vi "Measurement.vi"(0 "Position":T3(array[cluster]) {"Z" format="%.1f"; "Y" format="%.1f"; "X" format="%.1f"}, 1 "setup":T4=enum."Show Setup", 2 "Post Process":T2, 4 "File":T5, 5 "Results file":path, 7 "Raw data file":path, 11 "Setup filename":string) -> (14 "2nd plot":cluster{"X array":dbl[], "Y array":dbl[]}[](graph), 19 "Status Out":T1)   [LabVIEW 2013]
uses:
  Anemometry Sub Vis/Controls/Save_Data.ctl
  Anemometry Sub Vis/Controls/Setup.ctl
  Anemometry Sub Vis/Controls/Graph_Type.ctl
  Anemometry Sub Vis/Controls/Post_Process.ctl
  Anemometry Sub Vis/Gen Trav/Multi_Run_Status.ctl
  Anemometry Sub Vis/Controls/Inst_type.ctl
  ADAM Client/Sub VIs/ADAM Controls/Traverse_Level_State.ctl
  Anemometry Sub Vis/File/Setup_Filetype.ctl
  Anemometry Sub Vis/Globals/Trav_pos_global.vi
  Anemometry Sub Vis/Globals/Meas_global.vi
  Anemometry Sub Vis/Acquisition/PWA/PWAtasksGLOBAL.vi
  Anemometry Sub Vis/Acquisition/Data_Translation/DataTranslation_global.vi
  Anemometry Sub Vis/Globals/Preference_global.vi
  Anemometry Sub Vis/Globals/LDA_meas_global_1.vi
  Anemometry Sub Vis/Globals/LDA_meas_global_2.vi
  Anemometry Sub Vis/Globals/Dynamic_call_global.ph.vi
  Anemometry Sub Vis/Globals/Plug_in_data_global.vi
  Anemometry Sub Vis/Globals/Constants_global.vi
panel:
  out "Pause message":string
  out "Statistics":string[][](table)
  out "Actual Sampling freq":dbl=100.0 format="%.1f"
  in  "Desired Sampling freq (Hz)":dbl=100.0 format="%.1f"
  out "Current Block No":i32=5 caption="Current Block"
  in  "Pause":bool
  in  "No of Blocks":i32=5
  in  "stop":bool
  in  "No of samples":i32=1000 min=0 step=1
  in  "PP next block":bool
  in  "Tab Control":T6(tab)
  in  "Second Graph":T8={"Plot 1"=2, "Plot 2"=1, "Save graph"=0, "Plot Type"=enum."Vel histogram"} {"Save graph" items=["Do not save plot", "Save plot"]; "Plot 2" items=["Nothing", "U1", "U2", "Sync", "T", "WT1", "I1"]; "Plot 1" items=["Nothing", "U1", "U2", "Sync", "T", "WT1", "I1"]}
  in  "First Graph":T8={"Plot 1"=1, "Plot 2"=2, "Save graph"=0, "Plot Type"=enum."Velocity trace"} {"Save graph" items=["Do not save plot", "Save plot"]; "Plot 2" items=["Nothing", "U1", "U2", "Sync", "T", "WT1", "I1"]; "Plot 1" items=["Nothing", "U1", "U2", "Sync", "T", "WT1", "I1"]}
  out "First plot":cluster{"X array":dbl[], "Y array":dbl[]}[](graph)
  in  "Comments":string
  out "uv":dbl[][](graph)=[[-0.041806189081711534, -0.046435429052714985, -0.04035660097427599, -0.042187605126076694, -0.042052555599004206]]
  out "u^4":dbl[][](graph)
  out "u^3":dbl[][](graph)
  out "u^2":dbl[][](graph)=[[0.09743628875280319, 0.10575821456272283, 0.10126262927293661, 0.09890442087602569, 0.1022948212436432]]
  out "U":dbl[][](graph)=[[0.8295029456391334, 0.8915896983798417, 0.8415763502225625, 0.8394746126219594, 0.8466062785395404]]
  in  "Block average display control":cluster{"Name":string, "Include":bool}[](array[cluster])=[{"Name"="FF (C)", "Include"=FALSE}]
  in  "No of bins in histogram":i32=100
  out "Measurement time (min)":dbl=6.0 format="%.2f"
  in  "Correlate?":T9(ring)
  out "Diagnostic info":string[][](table)
  out "Array U":dbl[][](array[numeric]) format="%.2e"
  out "Array u^2":dbl[][](array[numeric]) format="%.2e"
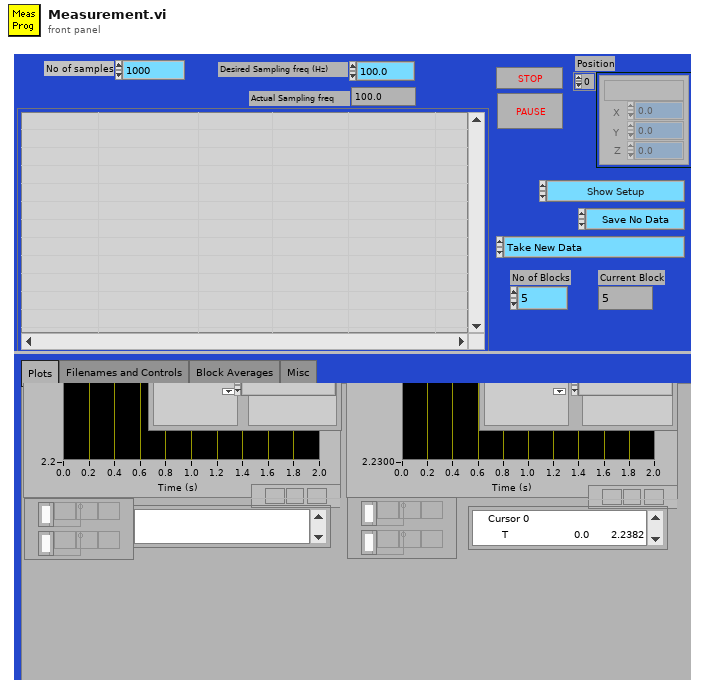
[diagram p1: front panel]
types:
  T1 = typedef "Multi_Run_Status.ctl" = enum16{"Continue", "Jump to Next Point", "Jump to Next Row", "Jump To Fall Back", "Terminate Run"}
  T2 = typedef "Post_Process.ctl" = enum16{"Take New Data", "Post Process Raw Data File"}
  T3 = cluster{"Name":string, "X":dbl, "Y":dbl, "Z":dbl}[]
  T4 = typedef "Setup.ctl" = enum16{"Run Program", "Show Setup", "Save Current Setup", "Setup Front Panel"}
  T5 = typedef "Save_Data.ctl" = enum16{"Save No Data", "Save Data"}
  T6 = enum32{"Plots", "Filenames and Controls", "Block Averages", "Misc"}
  T7 = typedef "Graph_Type.ctl" = enum16{"Show no graph", "Voltage trace", "Velocity trace", "Vel histogram", "Spectrum", "f.E(f) v Log f", "Auto-Corr"}
  T8 = cluster{"Plot 1":u16, "Plot 2":u16, "Save graph":u16, "Plot Type":T7}
  T9 = enum16{"Cross correlation off", "Show correlation panel", "Correlate without activating panel"}
  T10 = enum32{"Bad", "Idle", "Run top level", "Running"}
  T11 = cluster{"Name":string, "X":dbl, "Y":dbl, "Z":dbl}
  T12 = enum16{"Velocity", "Transit time", "Arrival time"}
  T13 = enum16{"Save no data", "Save data in new files", "Save data in existing files"}
  T14 = enum16{"Zero or one", "One", "Zero or more", "One or more"}
  T15 = cluster{"Weighting":dbl[], "Time (ms)":dbl[], "Voltage":dbl[], "Eng Values":dbl[]}
  T16 = typedef "Inst_type.ctl" = enum16{"Propeller anemometer", "Raw voltage", "Pressure Transducer", "Pitot-static tube", "Preston tube", "Hot wire", "Cross wire 1", "Cross wire 2", "Generic Linear", "Generic Polynomial", "Generic BackPoly", "Fast FID", "Thermocouple", "Cold wire", "Pulsed Wire", "LDA Vel", "LDA Tran time", "LDA Arr time"}
  T17 = typedef "Traverse_Level_State.ctl" = enum16{"Running", "Complete"}
  T18 = typedef "Setup_Filetype.ctl" = enum16{"Measurement Setups", "Calibration Setups", "General", "Results File Plotter Setups", "Speed Calib Tweaks"}
  T19 = typedef "Traverse_cluster.ctl" = cluster{"Start X":dbl, "Start Y":dbl, "Start Z":dbl, "End X":dbl, "End Y":dbl, "End Z":dbl, "No. of pts.":i32, "Spacing":T20, "Filename":path, "Tunnel Speed":dbl, "Averaging time (min)":dbl, "Extra Commands":string, "Specific Arguments":string, "Emission Rate (l/min)":dbl, "Trace Gas Concentration (%)":dbl, "Density Ratio":string, "Comments":string, "Row No":i32, "Row Type Selector":T21, "Completion time":string, "Row Duration (mins)":dbl, "No. of Valid pts.":i32, "Meas Setup File":string}
  T20 = typedef "Spacing.ctl" = enum16{"Linear", "Log", "Gauss", "Specified", "N/A"}
  T21 = typedef "Multi_run_mode.ctl" = enum16{"Move Traverse Only", "Set Tunnel Speed Only", "Set Source Only", "Set Measurement Conditions", "Single Measurement", "Vertical Profile", "Lateral Profile", "Longitudinal Profile", "Explore Volume", "Multi-Axis Profile", "Auto Calibrate", "Meas Fast FID Bkgnd", "Check Beam Power", "Scanning Valve Measurement", "Run VI Named:", "Set ADAM Ch", "Wait (minutes)", "Send Message", "Synchronize With:", "Fall Back to this Row", "Turn Off Row Repeating", "Blank Row", "Traverse 3D Volume"}
  T22 = typedef "Analysis_info_cluster.ctl" = cluster{"Colour":u32, "Inst type":T16, "Inst name":string, "Symbol":string, "Code name":string, "Extra Info":string, "Inst Array":T23, "Extra Titles":string[], "Extra Values":string[], "U":dbl, "u^2":dbl, "u^3":dbl, "u^4":dbl, "Skew_u":dbl, "Kurt_u":dbl, "Sd Error in Mean":dbl, "% u'/U":dbl, "X":dbl, "Y":dbl, "Z":dbl, "Timescale integral to 25%":dbl, "Sd Error in Variance":dbl, "Calib File":path, "Calib Constants":dbl[], "Output Position":bool, "Full Stats":bool, "Av Sampling Rate":dbl, "Av No of Samples":dbl, "Total Meas Time (s)":dbl, "ADAM Ch Name":string}
  T23 = typedef "Instrument_Array.ctl" = enum16{"PWA", "LDA", "Analogue"}
  T24 = typedef "LDA_Setup.ctl" = cluster{"dimensions":enum16{"1D", "2D"}, "Analogue Freq Multiplier":dbl}
  T25 = enum16{"Velocity", "Transit time", "Arrival time"}[]
  T26 = typedef "BSA_Type.ctl" = enum16{"57N11", "BSA F60"}
  T27 = typedef "BSA_info_Cluster.ctl" = cluster{"GPIB Address":string, "No of Check Bytes":i32, "Extra Info":string, "COLOUR":u32, "Wavelength (nm)":dbl}
  T28 = typedef "Ch_and_Spans.ctl" = cluster{"high limit (10V)":sgl, "low limit (-10V)":sgl, "Ch No":i16, "Var name":string, "Use Latest Calib":bool, "DAQmx Chan":tag}
  T29 = cluster{"Weighting":dbl[], "Time (ms)":dbl[], "Voltage":dbl[], "Eng Values":dbl[]}[]
  T30 = cluster{"Insts for plotting[0]":u16, "Insts for plotting[1]":u16}
  T31 = typedef "PWA_Data.ctl" = enum16{"No PWA Data", "One Ch PWA"}
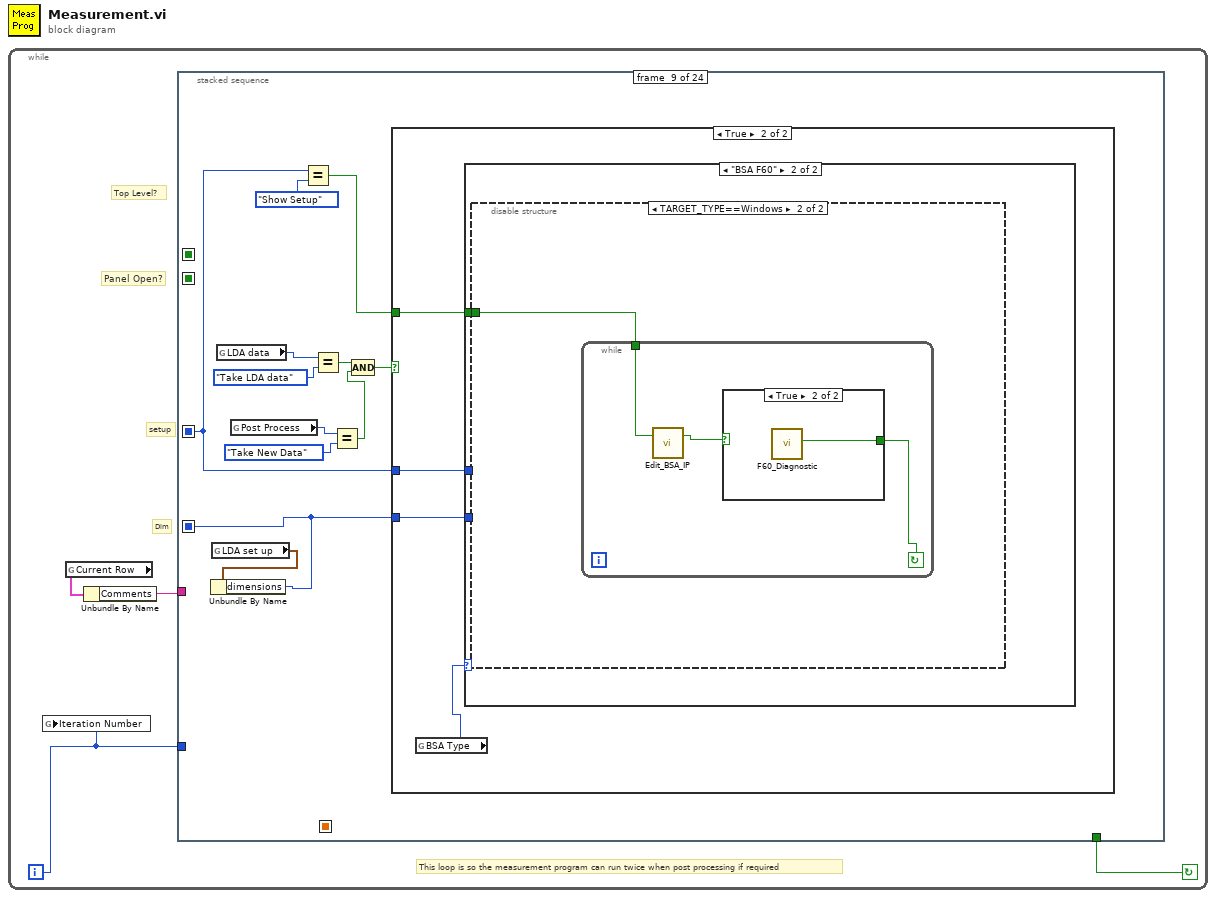
[diagram p0: block diagram]
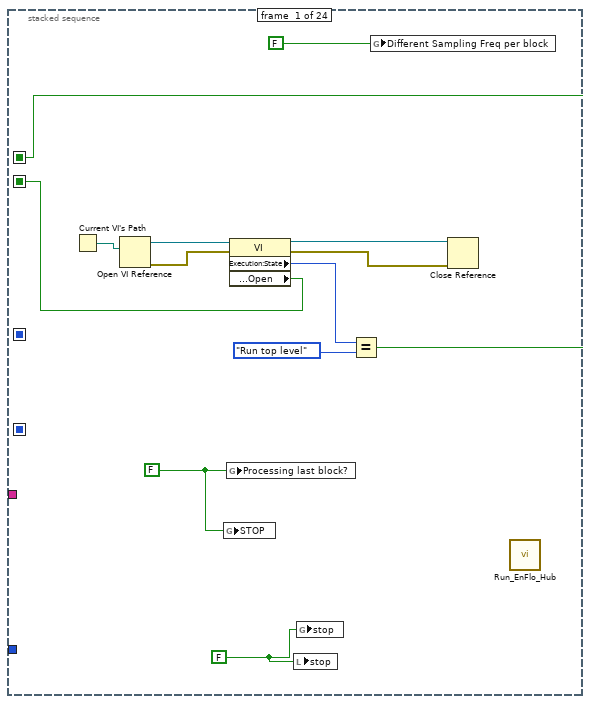
[diagram p2: hidden frame]
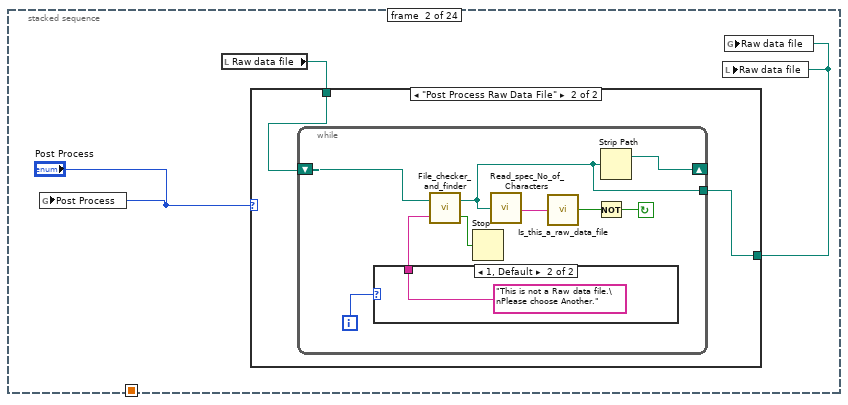
[diagram p3: hidden frame]
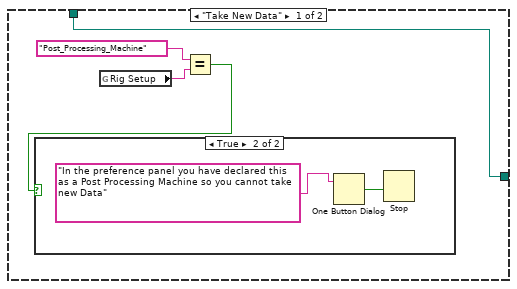
[diagram p4: hidden frame]
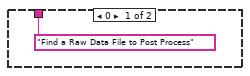
[diagram p6: hidden frame]
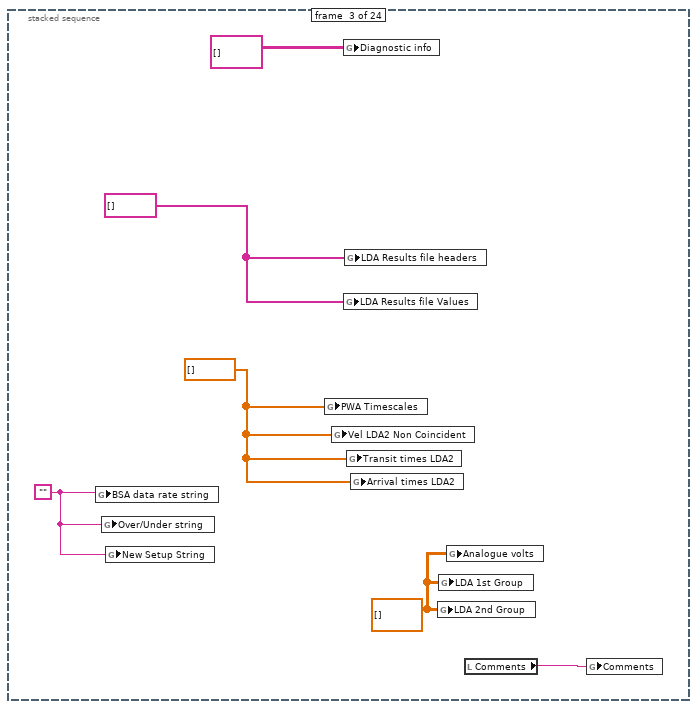
[diagram p7: hidden frame]
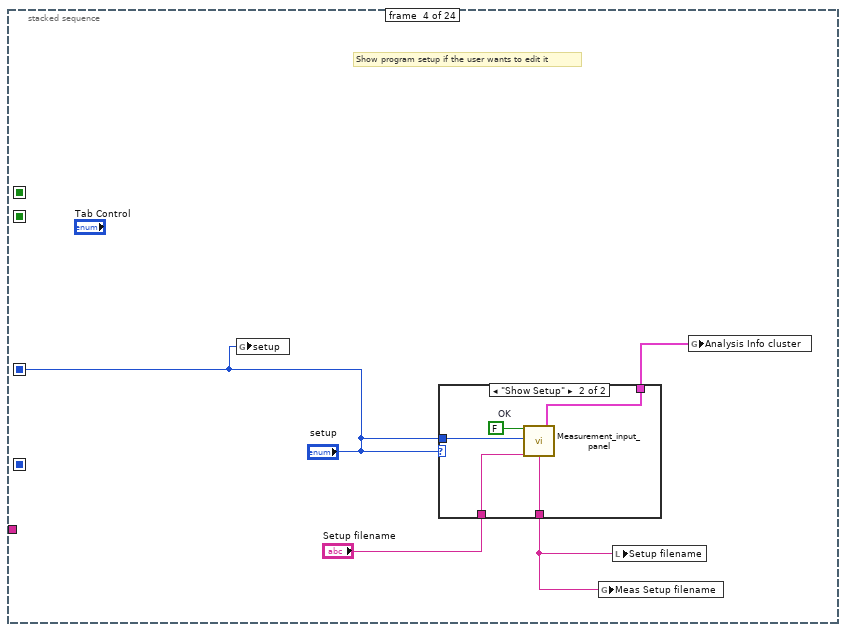
[diagram p8: hidden frame]
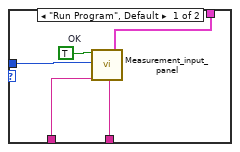
[diagram p9: hidden frame]
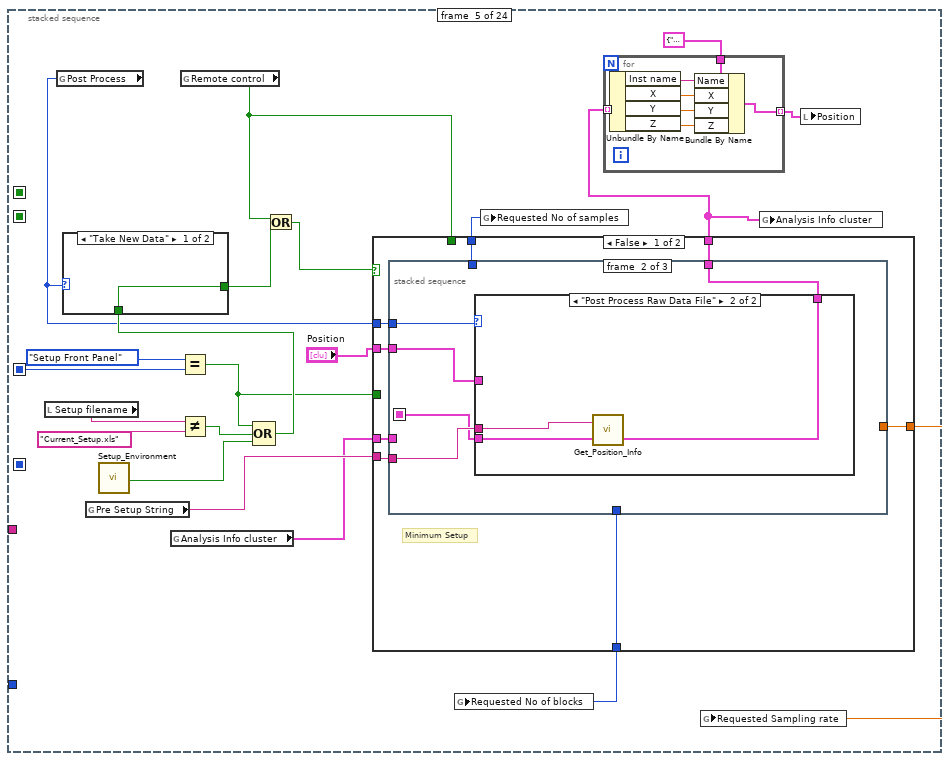
[diagram p10: hidden frame]
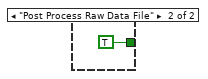
[diagram p11: hidden frame]
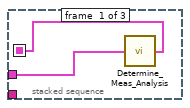
[diagram p12: hidden frame]
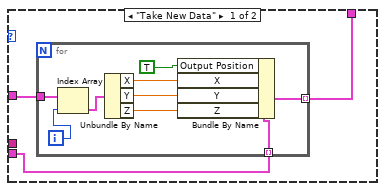
[diagram p13: hidden frame]
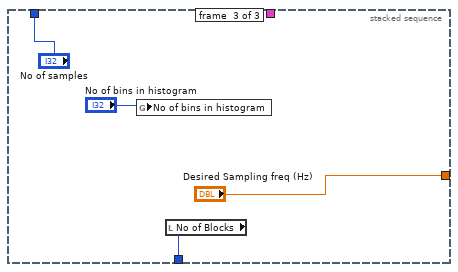
[diagram p14: hidden frame]
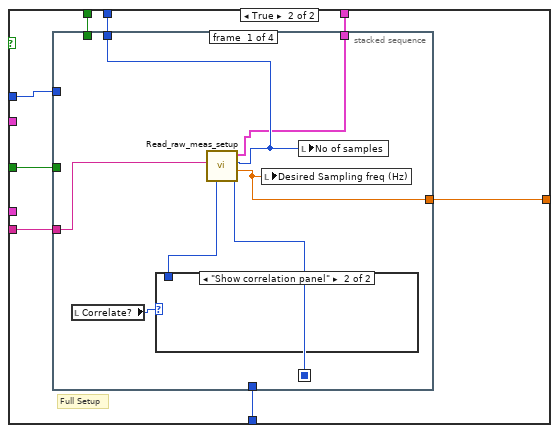
[diagram p15: hidden frame]
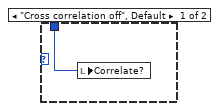
[diagram p16: hidden frame]
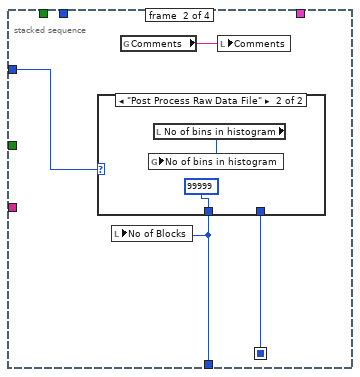
[diagram p17: hidden frame]
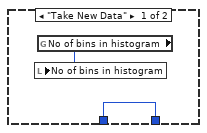
[diagram p18: hidden frame]
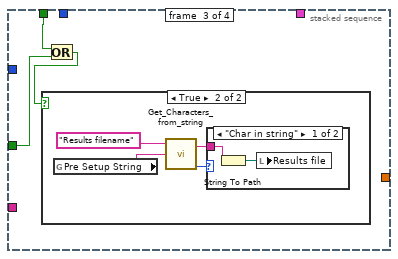
[diagram p19: hidden frame]
diagram:
  n1 = while {
    i -> [w1]
    stop <- w2 continue-if-true
    # "This loop is so the measurement program can run twice when post processing if required"
    # "Panel Open?"
    # "Top Level?"
    # "setup"
    # "Dim"
    n2 = global write "Meas_global.vi" "Iteration Number"(w1) -> ()
    n3 = global read "Trav_pos_global.vi" "Current Row"() -> (w3:T19)
    n4 = Unbundle By Name(w3) -> ("Comments"=w4:string)
    n5 = stacked-sequence {
      seq-local: [_ _ _ _ _ _ _ _ w207 _ _ _ _ _ _ _ _ _ _ _ _ _ _ _] -> [_ _ _ _ _ _ _ _ _ _ _ _ _ _ _ _ _ w750 _ _ _ _ _ _]
      seq-local: [_ _ _ "setup" _ _ _ _ _ _ _ _ _ _ _ _ _ _ _ _ _ _ _ _] -> [_ _ _ _ w71 _ _ _ w206 w287 _ _ _ _ w660 w680 w687 w751 w958 w1008 w1063 _ _ w1169]
      seq-local: [_ _ _ _ _ _ _ _ _ _ _ _ _ _ _ _ w683 _ _ _ _ _ _ _] -> [_ _ _ _ _ _ _ _ _ _ _ _ _ _ _ _ _ w749 w948 _ _ _ _ _]
      seq-local: [w7 _ _ _ _ _ _ _ _ _ _ _ _ _ _ _ _ _ _ _ _ _ _ _] -> [_ _ _ _ _ _ _ _ _ w267 _ _ _ _ w656 _ _ w748 _ _ _ _ _ _]
      seq-local: [w6 _ _ _ _ _ _ _ _ _ _ _ _ _ _ _ _ _ _ _ _ _ _ _] -> [_ _ _ _ _ _ _ _ _ _ _ _ w479 _ _ _ _ _ _ _ _ _ _ _]
      tunnel: w4 -> [_ _ _ _ _ _ _ w197 _ _ _ _ _ _ _ _ _ _ _ _ _ _ w1138 _]
      tunnel: w1 -> [_ _ _ _ _ _ _ _ _ _ _ _ _ _ _ _ _ _ _ _ _ _ w1133 _]
      tunnel: [_ _ _ _ _ _ _ _ _ _ _ _ _ _ _ _ _ _ _ _ _ _ w1132 _] -> w2
      frame #0 {
        w15 = FALSE ("Processing last block?")
        w16 = FALSE ("stop")
        n6 = Current VI's Path() -> (path=w8:path)
        n7 = Open VI Reference(vi path=w8) -> (vi reference=w9:refnum<vi>, error out=w10:errorcluster)  [unwired: 1 in, 4 out]
        n8 = global write "PWAtasksGLOBAL.vi" "STOP"(w15) -> ()
        n9 = global write "Meas_global.vi" "Processing last block?"(w15) -> ()
        n10 = property class="VI"(reference=w9, error in=w10) -> (reference out=w11:refnum<vi>, error out=w12:errorcluster, "Execution:State"=w13:T10, "Front Panel.Open"=w6:bool)
        n11 = local write "stop"(w16) -> ()
        n12 = global write "Meas_global.vi" "stop"(w16) -> ()
        n13 = Equal?(x=w13, y=T10."Run top level" ("Exec.State")) -> (x = y?=w7:bool)
        n14 = global write "DataTranslation_global.vi" "Different Sampling Freq per block"(FALSE ("Different Sampling Freq per block")) -> ()
        n15 = Close Reference(reference=w11, error in (no error)=w12) -> ()  [unwired: 1 out]
        n16 = call "Run_EnFlo_Hub.vi"() -> ()  [unwired: 8 out]
      }
      frame #1 {
        n17 = global write "Meas_global.vi" "Post Process"("Post Process") -> ()
        n18 = local read "Raw data file"() -> (w19:path)
        n19 = case shown="\"Post Process Raw Data File\"" "Post Process" {
          tunnel: [w23 w27] -> w18
          tunnel: w19 -> [w23 w26]
          frame "Take New Data" {
            n20 = global read "Preference_global.vi" "Rig Setup"() -> (w22:string)
            n21 = Equal?(x="Post_Processing_Machine" ("Rig Setup"), y=w22) -> (x = y?=w20:bool)
            n22 = case shown="True" w20 {
              frame False {
              }
              frame True {
                n23 = One Button Dialog(message="In the preference panel you have declared this as a Post Processing Machine so you cannot take new Data") -> (true=w24:bool)  [unwired: 1 in]
                n24 = Stop(stop? (T)=w24) -> ()
              }
            }
          }
          frame "Post Process Raw Data File" {
            n25 = while {
              tunnel: [w29] -> w27
              shift-left: w26 -> [w31]
              shift-right: [w30] -> _
              i -> [w32]
              stop <- w33 continue-if-true
              n26 = case shown="1, Default" w32 {
                tunnel: ["Find a Raw Data File to Post Process" ("Promp if not found") "This is not a Raw data file.\nPlease choose Another." ("Promp if not found")] -> w36
                frame 0 {
                }
                frame 1, Default {
                }
              }
              n27 = call "File_checker_and_finder.vi"("Promp if not found"=w36, "Filename In"=w31) -> ("cancelled"=w28:bool, "Filename Out"=w29:path)
              n28 = Stop(stop? (T)=w28) -> ()
              n29 = call "Read_spec_No_of_Characters.vi"("Filename"=w29) -> ("character string"=w35:string)  [unwired: 1 out]
              n30 = call "Is_this_a_raw_data_file.vi"("character string"=w35) -> ("Raw Dat File?"=w34:bool)  [unwired: 2 out]
              n31 = Not(x=w34) -> (.not. x?=w33:bool)
              n32 = Strip Path(path=w29) -> (stripped path=w30:path)  [unwired: 1 out]
            }
          }
        }
        n33 = local write "Raw data file"(w18) -> ()
        n34 = global write "Meas_global.vi" "Raw data file"(w18) -> ()
      }
      frame #2 {
        w39 = dbl[][] [] ("LDA 2nd Group")
        w40 = dbl[] [] ("LDA Timescales")
        w42 = string[] [] ("Plug in values")
        w44 = ""
        n35 = global write "Meas_global.vi" "BSA data rate string"(w44) -> ()
        n36 = global write "Meas_global.vi" "Over/Under string"(w44) -> ()
        n37 = global write "Meas_global.vi" "New Setup String"(w44) -> ()
        n38 = global write "PWAtasksGLOBAL.vi" "PWA Timescales"(w40) -> ()
        n39 = global write "LDA_meas_global_2.vi" "Vel LDA2 Non Coincident"(w40) -> ()
        n40 = global write "Meas_global.vi" "Diagnostic info"(string[][] [] ("Diagnostic info")) -> ()
        n41 = global write "LDA_meas_global_1.vi" "LDA Results file Values"(w42) -> ()
        n42 = global write "LDA_meas_global_1.vi" "LDA Results file headers"(w42) -> ()
        n43 = global write "LDA_meas_global_2.vi" "Transit times LDA2"(w40) -> ()
        n44 = global write "LDA_meas_global_2.vi" "Arrival times LDA2"(w40) -> ()
        n45 = global write "LDA_meas_global_2.vi" "LDA 2nd Group"(w39) -> ()
        n46 = global write "LDA_meas_global_2.vi" "LDA 1st Group"(w39) -> ()
        n47 = global write "Meas_global.vi" "Analogue volts"(w39) -> ()
        n48 = local read "Comments"() -> (w43:string)
        n49 = global write "Meas_global.vi" "Comments"(w43) -> ()
      }
      frame #3 {
        # "Show program setup if the user wants to edit it"
        n50 = global write "Meas_global.vi" "setup"("setup") -> ()
        n51 = case shown="\"Show Setup\"" "setup" {
          tunnel: [w52 w57] -> w48
          tunnel: "Setup filename" -> [w51 w56]
          tunnel: [w50 w55] -> w46
          tunnel: "setup" -> [w49 w54]
          frame "Run Program", Default {
            w53 = TRUE  # OK
            n52 = call "Measurement_input_panel.vi"("OK"=w53, "setup"=w49, "Setup filename"=w51) -> ("Setup filename out"=w50:string, "Analysis Info cluster"=w52:T22[])  [unwired: 15 out]
          }
          frame "Show Setup" {
            w58 = FALSE  # OK
            n53 = call "Measurement_input_panel.vi"("OK"=w58, "setup"=w54, "Setup filename"=w56) -> ("Setup filename out"=w55:string, "Analysis Info cluster"=w57:T22[])  [unwired: 15 out]
          }
        }
        n54 = global write "Meas_global.vi" "Meas Setup filename"(w46) -> ()
        n55 = local write "Setup filename"(w46) -> ()
        n56 = global write "Meas_global.vi" "Analysis Info cluster"(w48) -> ()
      }
      frame #4 {
        n57 = local read "Setup filename"() -> (w75:string)
        n58 = global read "Meas_global.vi" "Post Process"() -> (w70:T2)
        n59 = global read "Meas_global.vi" "Pre Setup String"() -> (w66:string)
        n60 = call "Setup_Environment.vi"() -> ("First Time"=w67:bool)  [unwired: 1 in]
        n61 = global read "Meas_global.vi" "Analysis Info cluster"() -> (w63:T22[])
        n62 = Equal?(x=Setup."Setup Front Panel" ("setup"), y=w71) -> (x = y?=w64:bool)
        n63 = Not Equal?(x=w75, y="Current_Setup.xls" ("Setup filename")) -> (x != y?=w73:bool)
        n64 = global read "Meas_global.vi" "Remote control"() -> (w65:bool)
        n65 = Compound Arithmetic op=OR(w64, w73, w67) -> (w72:bool)
        n66 = case shown="\"Take New Data\"" w70 {
          tunnel: [w87 TRUE] -> w79
          tunnel: w72 -> [w87 _]
          frame "Take New Data" {
          }
          frame "Post Process Raw Data File" {
          }
        }
        n67 = Or(x=w65, y=w79) -> (x .or. y?=w78:bool)
        n68 = case shown="False" w78 {
          tunnel: w70 -> [w92 w130]
          tunnel: [w96 w129] -> w68
          tunnel: [w95 w124] -> w77
          tunnel: [w94 w128] -> w76
          tunnel: [w93 w127] -> w62
          tunnel: w66 -> [w91 w126]
          tunnel: "Position" -> [w90 _]
          tunnel: w65 -> [_ w125]
          tunnel: w64 -> [_ w123]
          tunnel: w63 -> [w89 _]
          frame False {
            # "Minimum Setup"
            n69 = stacked-sequence {
              seq-local: [w97 _ _] -> [_ w99 _]
              tunnel: [_ _ "Desired Sampling freq (Hz)"] -> w96
              tunnel: [_ _ w121] -> w95
              tunnel: [_ _ "No of samples"] -> w94
              tunnel: [_ w102 _] -> w93
              tunnel: w92 -> [_ w103 _]
              tunnel: w91 -> [_ w101 _]
              tunnel: w90 -> [_ w100 _]
              tunnel: w89 -> [w98 _ _]
              frame #0 {
                n70 = call "Determine_Meas_Analysis.vi"("Analysis info Cluster In"=w98) -> ("Analysis info Cluster Out"=w97:T22[])
              }
              frame #1 {
                n71 = case shown="\"Post Process Raw Data File\"" w103 {
                  tunnel: [w104 w116] -> w102
                  tunnel: w100 -> [w106 _]
                  tunnel: w101 -> [_ w117]
                  tunnel: w99 -> [w105 w118]
                  frame "Take New Data" {
                    n72 = for {
                      tunnel: w106 -> [w109]
                      tunnel: w105 -> [w115] mode=indexing
                      tunnel: [w111] -> w104 mode=indexing
                      i -> [w110]
                      n73 = Index Array(array=w109, index=w110) -> (element=w108:T11)
                      n74 = Unbundle By Name(w108) -> ("X"=w112:dbl, "Y"=w113:dbl, "Z"=w114:dbl)
                      n75 = Bundle By Name(cluster=w115, "Output Position"=TRUE, "X"=w112, "Y"=w113, "Z"=w114) -> (w111:T22)
                    }
                  }
                  frame "Post Process Raw Data File" {
                    n76 = call "Get_Position_Info.vi"("Analysis Info cluster"=w118, "Setup file string"=w117) -> ("Analysis Info cluster 2"=w116:T22[])  [unwired: 1 in]
                  }
                }
              }
              frame #2 {
                n77 = global write "Meas_global.vi" "No of bins in histogram"("No of bins in histogram") -> ()
                n78 = local read "No of Blocks"() -> (w121:i32)
              }
            }
          }
          frame True {
            # "Full Setup"
            n79 = stacked-sequence {
              seq-local: [w134 _ _ _] -> [_ w140 _ _]
              tunnel: w130 -> [_ w141 _ w156]
              tunnel: [w137 _ _ _] -> w129
              tunnel: [w136 _ _ _] -> w128
              tunnel: [w133 _ _ _] -> w127
              tunnel: w126 -> [w135 _ _ _]
              tunnel: w125 -> [_ _ w149 _]
              tunnel: [_ w139 _ _] -> w124
              tunnel: w123 -> [_ _ w148 _]
              frame #0 {
                n80 = local read "Correlate?"() -> (w132:T9)
                n81 = call "Read_raw_meas_setup.vi"("Setup file string"=w135) -> ("No of Blocks"=w134:i32, "Sampling freq (Hz)"=w137:dbl, "No of samples"=w136:i32, "Analysis Info cluster 2"=w133:T22[], "Correlate?"=w131:T9)  [unwired: 4 out]
                n82 = case shown="\"Show correlation panel\"" w132 {
                  tunnel: w131 -> [w138 _]
                  frame "Cross correlation off", Default {
                    n83 = local write "Correlate?"(w138) -> ()
                  }
                  frame "Show correlation panel" {
                  }
                }
                n84 = local write "Desired Sampling freq (Hz)"(w137) -> ()
                n85 = local write "No of samples"(w136) -> ()
              }
              frame #1 {
                n86 = case shown="\"Post Process Raw Data File\"" w141 {
                  tunnel: [w144 99999 ("No of Blocks")] -> w139
                  tunnel: w140 -> [w144 _]
                  frame "Take New Data" {
                    n87 = global read "Meas_global.vi" "No of bins in histogram"() -> (w143:i32)
                    n88 = local write "No of bins in histogram"(w143) -> ()
                  }
                  frame "Post Process Raw Data File" {
                    n89 = local read "No of bins in histogram"() -> (w145:i32)
                    n90 = global write "Meas_global.vi" "No of bins in histogram"(w145) -> ()
                  }
                }
                n91 = local write "No of Blocks"(w139) -> ()
                n92 = global read "Meas_global.vi" "Comments"() -> (w142:string)
                n93 = local write "Comments"(w142) -> ()
              }
              frame #2 {
                n94 = Or(x=w149, y=w148) -> (x .or. y?=w147:bool)
                n95 = case shown="True" w147 {
                  frame False {
                  }
                  frame True {
                    n96 = global read "Meas_global.vi" "Pre Setup String"() -> (w150:string)
                    n97 = call "Get_Characters_from_string.vi"("Input string"=w150, "Variable name"="Results filename") -> ("Status"=w153:enum16{"Char in string", "Char not in string"}, "Value"=w152:string)  [unwired: 1 in]
                    n98 = case shown="\"Char in string\"" w153 {
                      tunnel: w152 -> [w155 _]
                      frame "Char in string" {
                        n99 = String To Path(string=w155) -> (path=w154:path)
                        n100 = local write "Results file"(w154) -> ()
                      }
                      frame "Char not in string" {
                      }
                    }
                  }
                }
              }
              frame #3 {
                n101 = case shown="\"Take New Data\"" w156 {
                  frame "Take New Data" {
                    n102 = global read "Meas_global.vi" "Second Graph"() -> (w157:T8)
                    n103 = global read "Meas_global.vi" "First Graph"() -> (w158:T8)
                    n104 = local write "Second Graph"(w157) -> ()
                    n105 = local write "First Graph"(w158) -> ()
                  }
                  frame "Post Process Raw Data File" {
                  }
                }
              }
            }
          }
        }
        n106 = global write "Meas_global.vi" "Requested No of blocks"(w77) -> ()
        n107 = global write "Meas_global.vi" "Requested No of samples"(w76) -> ()
        n108 = for {
          tunnel: w62 -> [w86] mode=indexing
          tunnel: [w82] -> w60 mode=indexing
          tunnel: T11 {"Name"="", "X"=0.0, "Y"=0.0, "Z"=0.0} ("Position") -> [w81]
          n109 = Unbundle By Name(w86) -> ("Inst name"=w80:string, "X"=w83:dbl, "Y"=w84:dbl, "Z"=w85:dbl)
          n110 = Bundle By Name(cluster=w81, "Name"=w80, "X"=w83, "Y"=w84, "Z"=w85) -> (w82:T11)
        }
        n111 = global write "Meas_global.vi" "Requested Sampling rate"(w68) -> ()
        n112 = global write "Meas_global.vi" "Analysis Info cluster"(w62) -> ()
        n113 = local write "Position"(w60) -> ()
      }
      frame #5 {
        n114 = global read "Meas_global.vi" "Post Process"() -> (w159:T2)
        n115 = case shown="\"Post Process Raw Data File\"" w159 {
          tunnel: [w162 w163] -> w160
          frame "Take New Data" {
            n116 = Get Date/Time In Seconds() -> (seconds since 1Jan1904=w161:timestamp)
            n117 = To Double Precision Float(number=w161) -> (double precision float=w162:dbl)
          }
          frame "Post Process Raw Data File" {
            n118 = global read "Meas_global.vi" "Pre Setup String"() -> (w166:string)
            n119 = call "Get_Characters_from_string.vi"("Input string"=w166, "Variable name"="Seconds since 1/1/04") -> ("Value"=w164:string)  [unwired: 1 in, 1 out]
            n120 = call "String_2_Number.vi"("Value"=w164) -> ("Numeric"=w163:dbl)
          }
        }
        n121 = global write "Meas_global.vi" "Time Data was Aquired"(w160) -> ()
      }
      frame #6 {
        n122 = global read "Dynamic_call_global.ph.vi" "Initial Plug Ins"() -> (w168:string[])
        n123 = global read "Dynamic_call_global.ph.vi" "Initial Plug Ins Extra"() -> (w169:string[])
        n124 = Build Array (concatenate)(w169, w168) -> (w167:string[])
        n125 = Array Size(array=w167) -> (size(s)=w171:i32)
        n126 = Greater Than 0?(x=w171) -> (x > 0?=w170:bool)
        n127 = case shown="True" w170 {
          tunnel: w167 -> [_ w172]
          frame False {
          }
          frame True {
            n128 = stacked-sequence {
              tunnel: w172 -> [w174 _]
              frame #0 {
                n129 = global read "Meas_global.vi" "Post Process"() -> (w176:T2)
                n130 = call "Plug_in_Directories.vi"() -> ("Initial"=w173:path)  [unwired: 3 out]
                n131 = Equal?(x=w176, y=Post_Process."Post Process Raw Data File" ("Post Process")) -> (x = y?=w175:bool)
                n132 = for {
                  tunnel: w175 -> [w182]
                  tunnel: w174 -> [w179] mode=indexing
                  tunnel: w173 -> [w178]
                  w189 = FALSE  # Dialog Box (T)
                  n133 = Build Path(base path=w178, name or relative path=w179) -> (appended path=w180:path)
                  n134 = Open VI Reference(vi path=w180) -> (vi reference=w187:refnum<vi>, error out=w186:errorcluster)  [unwired: 2 in, 3 out]
                  n135 = property class="VI"(reference=w187, error in=w186, "Front Panel Window:Open"=TRUE ("Wait until done")) -> (reference out=w185:refnum<vi>, error out=w184:errorcluster)
                  n136 = invoke class="VI" method="Run VI"(reference=w185, error in=w184, "Wait until done"=w182, "Auto Dispose Ref"=FALSE) -> (reference out=w192:refnum<vi>, error out=w191:errorcluster)  [unwired: 1 in, 3 out]
                  n137 = Close Reference(reference=w192, error in (no error)=w191) -> (error out=w190:errorcluster)
                  n138 = call "EnFlo_Error_Handler.vi"("error in (no error)"=w190, "Error Type"="Launching Initial Plug In", "Dialog Box (T)"=w189) -> ()  [unwired: 3 out]
                }
              }
              frame #1 {
                n139 = global read "Meas_global.vi" "Requested No of blocks"() -> (w194:i32)
                n140 = global read "Meas_global.vi" "Comments"() -> (w193:string)
                n141 = local write "Comments"(w193) -> ()
                n142 = local write "No of Blocks"(w194) -> ()
              }
            }
          }
        }
      }
      frame #7 {
        n143 = local read "Comments"() -> (w198:string)
        n144 = Concatenate Strings(w197, w198) -> (w196:string)
        n145 = call "Text_without_format.vi"("Input string"=w196) -> ("Output string"=w195:string)
        n146 = local write "Comments"(w195) -> ()
        n147 = global write "Meas_global.vi" "Comments"(w195) -> ()
      }
      frame #8 {
        n148 = global read "Meas_global.vi" "LDA set up"() -> (w208:T24)
        n149 = Unbundle By Name(w208) -> ("dimensions"=w207:enum16{"1D", "2D"})
        n150 = global read "Meas_global.vi" "LDA data"() -> (w203:enum16{"No LDA data", "Take LDA data"})
        n151 = global read "Meas_global.vi" "Post Process"() -> (w200:T2)
        n152 = Equal?(x=w206, y=Setup."Show Setup" ("setup")) -> (x = y?=w209:bool)
        n153 = Equal?(x=w203, y=enum16{"No LDA data", "Take LDA data"}."Take LDA data" ("LDA data")) -> (x = y?=w204:bool)
        n154 = Equal?(x=w200, y=Post_Process."Take New Data" ("Post Process")) -> (x = y?=w201:bool)
        n155 = Compound Arithmetic op=AND(w204, w201) -> (w205:bool)
        n156 = case shown="True" w205 {
          tunnel: w207 -> [_ w219]
          tunnel: w206 -> [_ w218]
          tunnel: w209 -> [_ w216]
          frame False {
            n157 = Build Array(T12."Velocity", T12."Transit time", T12."Arrival time") -> (w211:T25)
            n158 = global write "LDA_meas_global_1.vi" "Number of measured quantities"(3 ("Number of measured quantities")) -> ()
            n159 = global write "LDA_meas_global_2.vi" "data type"(w211) -> ()
            n160 = global write "LDA_meas_global_1.vi" "data type"(w211) -> ()
          }
          frame True {
            n161 = global read "LDA_meas_global_1.vi" "BSA Type"() -> (w217:T26)
            n162 = case shown="\"BSA F60\"" w217 {
              tunnel: w219 -> [w221 _]
              tunnel: w218 -> [w220 _]
              tunnel: w216 -> [_ w257]
              frame "57N11" {
                n163 = stacked-sequence {
                  tunnel: w221 -> [w224 w250]
                  tunnel: w220 -> [w223 _]
                  frame #0 {
                    n164 = global read "Meas_global.vi" "Remote control"() -> (w222:bool)
                    n165 = case shown="\"2D\"" w224 {
                      tunnel: w223 -> [w226 w239]
                      tunnel: w222 -> [w225 w238]
                      frame "2D" {
                        n166 = while {
                          tunnel: w225 -> [w227]
                          tunnel: w226 -> [w228]
                          stop <- w229 continue-if-true
                          n167 = stacked-sequence {
                            tunnel: [_ _ w235] -> w229
                            tunnel: w228 -> [w230 w232 _]
                            tunnel: w227 -> [_ _ w234]
                            frame #0 {
                              w231 = "1"  # BSA Number
                              n168 = call "Control_BSA_setup.vi"("setup"=w230, "BSA number"=w231) -> ()  [unwired: 14 out]
                            }
                            frame #1 {
                              w233 = "2"  # BSA Number
                              n169 = call "Control_BSA_setup.vi"("setup"=w232, "BSA number"=w233) -> ()  [unwired: 14 out]
                            }
                            frame #2 {
                              n170 = case shown="False" w234 {
                                tunnel: [w236 FALSE ("ok")] -> w235
                                frame False {
                                n171 = call "BSA_setup_check.vi"() -> ("ok"=w236:bool)
                                }
                                frame True {
                                }
                              }
                            }
                          }
                        }
                      }
                      frame "1D" {
                        n172 = stacked-sequence {
                          tunnel: w239 -> [w240 _]
                          tunnel: w238 -> [_ _]
                          frame #0 {
                            w241 = "1"  # BSA Number
                            n173 = call "Control_BSA_setup.vi"("setup"=w240, "BSA number"=w241) -> ()  [unwired: 14 out]
                          }
                          frame #1 {
                            n174 = global read "LDA_meas_global_2.vi" "BSA2 info"() -> (w242:T27)
                            n175 = Unbundle By Name(w242) -> ("GPIB Address"=w243:string)
                            n176 = call "Set_BSA_Coincidence.vi"("GPIB address"=w243, "Set Coincidence"=enum16{"Slave", "Master", "Private"}."Slave") -> ()  [unwired: 1 in, 5 out]
                          }
                        }
                      }
                    }
                  }
                  frame #1 {
                    n177 = global read "Meas_global.vi" "Remote control"() -> (w248:bool)
                    n178 = Equal?(x=w250, y=enum16{"1D", "2D"}."2D" ("dimensions")) -> (x = y?=w246:bool)
                    n179 = Not(x=w248) -> (.not. x?=w247:bool)
                    n180 = And(x=w247, y=w246) -> (x .and. y?=w245:bool)
                    n181 = case shown="True" w245 {
                      frame False {
                      }
                      frame True {
                        n182 = global read "LDA_meas_global_1.vi" "BSA1 info"() -> (w252:T27)
                        n183 = global read "LDA_meas_global_2.vi" "BSA2 info"() -> (w253:T27)
                        n184 = Build Array(w252, w253) -> (w251:T27[])
                        n185 = for {
                          tunnel: w251 -> [w255] mode=indexing
                          n186 = Unbundle By Name(w255) -> ("GPIB Address"=w254:string)
                          n187 = call "Set_BSA_Coincidence.vi"("GPIB address"=w254, "Set Coincidence"=enum16{"Slave", "Master", "Private"}."Master") -> ()  [unwired: 1 in, 5 out]
                        }
                      }
                    }
                  }
                }
              }
              frame "BSA F60" {
                n188 = disable-structure shown="TARGET_TYPE==Windows" {
                  disable-tunnel: w257 -> [_ w258]
                  frame condition #0 {
                  }
                  frame condition #1 (active) {
                    n189 = while {
                      tunnel: w258 -> [w261]
                      stop <- w259 continue-if-true
                      n190 = call "Edit_BSA_IP.vi"("Show Panel"=w261) -> ("Run LDA Diagnostic Out"=w260:bool)  [unwired: 2 out]
                      n191 = case shown="True" w260 {
                        tunnel: [FALSE w263] -> w259
                        frame False {
                        }
                        frame True {
                          n192 = call "F60_Diagnostic.vi"() -> ("Edit BSA Setup Out"=w263:bool)  [unwired: 11 in]
                        }
                      }
                    }
                  }
                }
              }
            }
          }
        }
      }
      frame #9 {
        w272 = Save_Data."Save No Data" ("File")
        w288 = Post_Process."Take New Data"  # Post Process
        n193 = global read "Trav_pos_global.vi" "Meas Setup Number"() -> (w268:i32)
        n194 = Not Equal?(x=Setup."Run Program" ("setup"), y=w287) -> (x != y?=w273:bool)
        n195 = call "Current_Filepath.vi"("Filename in"="Results file", "Data Type"="Results") -> ("Filename Out"=w266:path)  [unwired: 1 out]
        n196 = global read "Meas_global.vi" "Remote control"() -> (w284:bool)
        n197 = global read "Meas_global.vi" "Post Process"() -> (w275:T2)
        n198 = Equal?(x="File", y=w272) -> (x = y?=w282:bool)
        n199 = case shown="1, Default" w268 {
          tunnel: [w291 w293] -> w269
          tunnel: w266 -> [w291 w300]
          tunnel: w268 -> [_ w301]
          frame 0 {
          }
          frame 1, Default {
            n200 = Add(x=96, y=w301) -> (x+y=w303:i32)
            n201 = Build Array(w303) -> (w304:i32[])
            n202 = Strip Path(path=w300) -> (stripped path=w294:path, name=w299:string)
            n203 = Byte Array To String(unsigned byte array=w304) -> (string=w297:string)
            n204 = call "Add_filename_suffix.vi"("Filename"=w299) -> ("Original Suffix"=w296:string, "Base name"=w298:string)  [unwired: 1 in, 2 out]
            n205 = Format Into String(format string="%s_%s%s", w298, w297, w296) -> (resulting string=w295:string)  [unwired: 2 in, 1 out]
            n206 = Build Path(base path=w294, name or relative path=w295) -> (appended path=w293:path)
          }
        }
        n207 = Equal?(x=w275, y=w288) -> (x = y?=w274:bool)
        n208 = And(x=w284, y=w274) -> (x .and. y?=w280:bool)
        n209 = Compound Arithmetic op=AND(w282, invert w284, w274, invert w273) -> (w283:bool)
        n210 = while {
          shift-left: _ -> [w309]
          shift-right: [w306] -> _
          tunnel: "File" -> [w307]
          tunnel: [w310] -> w281
          tunnel: w283 -> [w306]
          stop <- FALSE continue-if-true
          n211 = Compound Arithmetic op=AND(w306, invert w309) -> (w308:bool)
          n212 = case shown="True" w308 {
            tunnel: [w311 w314] -> w310
            tunnel: w307 -> [w311 _]
            frame False {
            }
            frame True {
              n213 = Two Button Dialog(message="Do you wish to save the data?", 1:"Save Data" ("F button name (\"Cancel\")"), 2:"Save No Data" ("T button name (\"OK\")")) -> (T button?=w315:bool)
              n214 = Select(t=Save_Data."Save No Data" ("File"), s=w315, f=Save_Data."Save Data" ("File")) -> (s? t:f=w314:T5)
            }
          }
        }
        n215 = Equal?(x=w272, y=w281) -> (x = y?=w271:bool)
        n216 = Or(x=w271, y=w273) -> (x .or. y?=w286:bool)
        n217 = case shown="False" w286 {
          tunnel: w269 -> [w330 w338]
          tunnel: [w329 w338] -> w289
          tunnel: "Raw data file" -> [w328 w339]
          tunnel: [w323 w339] -> w278
          tunnel: w287 -> [w327 _]
          tunnel: w281 -> [w326 _]
          tunnel: [w324 T13."Save no data" ("File output")] -> w276
          tunnel: [w325 w336] -> w270
          tunnel: w280 -> [_ w333]
          tunnel: w273 -> [_ w332]
          tunnel: w267 -> [w322 _]
          frame False {
            n218 = call "File_setup.vi"("Measurement is top level?"=w322, "Results file"=w330, "Raw data file"=w328, "setup"=w327, "File"=w326) -> ("Results file output"=w329:path, "Raw data file output"=w323:path, "Raw data option"=w325:enum16{"Save raw data", "Raw data not saved"}, "File output"=w324:T13)
          }
          frame True {
            w334 = enum16{"Save raw data", "Raw data not saved"}."Raw data not saved"  # Raw data option
            n219 = global read "Meas_global.vi" "Raw data option"() -> (w335:enum16{"Save raw data", "Raw data not saved"})
            n220 = Compound Arithmetic op=AND(w333, invert w332) -> (w331:bool)
            n221 = Select(t=w335, s=w331, f=w334) -> (s? t:f=w336:enum16{"Save raw data", "Raw data not saved"})
          }
        }
        n222 = case shown="\"Save raw data\"" w270 {
          tunnel: w278 -> [w319 w321]
          tunnel: [w319 w320] -> w277
          frame "Raw data not saved" {
          }
          frame "Save raw data" {
            n223 = call "Find_Unique_Filename.vi"("Path In"=w321) -> ("Unique Path Out"=w320:path)  [unwired: 1 in, 1 out]
          }
        }
        n224 = local write "Results file"(w289) -> ()
        n225 = global write "Meas_global.vi" "Results file"(w289) -> ()
        n226 = global write "Meas_global.vi" "Raw data option"(w270) -> ()
        n227 = global write "Meas_global.vi" "File"(w276) -> ()
        n228 = global write "Meas_global.vi" "Raw data file"(w277) -> ()
        n229 = local write "Raw data file"(w277) -> ()
        n230 = local write "File"(w281) -> ()
      }
      frame #10 {
        n231 = global read "Meas_global.vi" "Ch & spans"() -> (w341:T28[])
        n232 = local read "Block average display control"() -> (w344:cluster{"Name":string, "Include":bool}[])
        n233 = global read "Meas_global.vi" "Analysis Info cluster"() -> (w340:T22[])
        n234 = global write "Meas_global.vi" "Ch & spans + mod limits"(w341) -> ()
        n235 = for {
          tunnel: w340 -> [w352] mode=indexing
          tunnel: w344 -> [w351]
          tunnel: [w347] -> w343 mode=indexing
          tunnel: [w348] -> w342 mode=indexing
          i -> [w350]
          n236 = Unbundle By Name(w352) -> ("Symbol"=w347:string)
          n237 = Index Array(array=w351, index=w350) -> (element=w349:cluster{"Name":string, "Include":bool})
          n238 = Bundle By Name(cluster=w349, "Name"=w347) -> (w348:cluster{"Name":string, "Include":bool})
        }
        n239 = local write "Block average display control"(w342) -> ()
        n240 = Build Array (concatenate)("Nothing", w343) -> (w345:string[])
        n241 = property on="Plot 1" class="Ring (strict)"("Strings []"=w345) -> ()  [unwired: 2 in, 2 out]
        n242 = property on="Plot 1" class="Ring (strict)"("Strings []"=w345) -> ()  [unwired: 2 in, 2 out]
        n243 = property on="Plot 2" class="Ring (strict)"("Strings []"=w345) -> ()  [unwired: 2 in, 2 out]
        n244 = property on="Plot 2" class="Ring (strict)"("Strings []"=w345) -> ()  [unwired: 2 in, 2 out]
      }
      frame #11 {
        n245 = global read "Meas_global.vi" "Analysis Info cluster"() -> (w355:T22[])
        n246 = for {
          tunnel: w355 -> [w476] mode=indexing
          tunnel: [w475] -> w356
          stop <- w475 stop-if-true
          n247 = Unbundle By Name(w476) -> ("Inst type"=w477:T16)
          n248 = Equal?(x=w477, y=Inst_type."LDA Vel" ("Inst type")) -> (x = y?=w475:bool)
        }
        n249 = global read "Meas_global.vi" "Post Process"() -> (w359:T2)
        n250 = Equal?(x=w359, y=Post_Process."Post Process Raw Data File" ("Post Process")) -> (x = y?=w357:bool)
        n251 = And(x=w356, y=w357) -> (x .and. y?=w353:bool)
        n252 = stacked-sequence {
          seq-local: [w361 _ _ _] -> [_ w389 w445 _]
          seq-local: [_ w391 _ _] -> [_ _ w444 _]
          seq-local: [w360 _ _ _] -> [_ w388 _ _]
          tunnel: w355 -> [w364 w392 _ w474]
          tunnel: w353 -> [_ w393 _ _]
          tunnel: "Correlate?" -> [_ w390 _ _]
          frame #0 {
            w362 = "RV (WT"
            n253 = String Length(string=w362) -> (length=w363:i32)
            n254 = for {
              tunnel: w364 -> [w383] mode=indexing
              shift-right: [w373] -> w365
              shift-left: i32[] [] -> [w374]
              tunnel: w363 -> [w371]
              tunnel: w362 -> [w369]
              tunnel: [w367] -> w360 mode=indexing
              i -> [w375]
              n255 = Unbundle By Name(w383) -> ("Inst name"=w367:string, "Symbol"=w382:string, "Code name"=w380:string)
              n256 = String Subset(string=w367, length (rest)=w371) -> (substring=w370:string)  [unwired: 1 in]
              n257 = Match Pattern(string=w380, regular expression="Derived") -> (offset past match=w379:i32)  [unwired: 1 in, 3 out]
              n258 = Not Equal?(x=w369, y=w370) -> (x != y?=w368:bool)
              n259 = Less Than 0?(x=w379) -> (x < 0?=w378:bool)
              n260 = Not Equal?(x="Sync", y=w382) -> (x != y?=w377:bool)
              n261 = Compound Arithmetic op=AND(w368, w377, w378) -> (w376:bool)
              n262 = case shown="True" w376 {
                tunnel: w375 -> [_ w387]
                tunnel: w374 -> [w384 w386]
                tunnel: [w384 w385] -> w373
                frame False {
                }
                frame True {
                  n263 = Build Array (concatenate)(w386, w387) -> (w385:i32[])
                }
              }
            }
            n264 = call "Chs_to_Correlate.vi"("Valid Ch to correlate"=w365) -> ("Correlation Pairs"=w361:i32[][])
          }
          frame #1 {
            n265 = case shown="False" w393 {
              tunnel: w392 -> [_ _]
              tunnel: [w394 w441] -> w391
              tunnel: w390 -> [w400 _]
              tunnel: w389 -> [w395 w441]
              tunnel: w388 -> [w401 _]
              frame False {
                n266 = global read "Meas_global.vi" "correlate"() -> (w398:i32[][])
                n267 = for {
                  tunnel: w395 -> [w426] mode=indexing
                  tunnel: w401 -> [w431]
                  tunnel: [w422] -> w399 mode=indexing
                  tunnel: w398 -> [w427]
                  shift-right: [w423] -> w396
                  shift-left: string[] [] -> [w424]
                  n268 = Index Array(array=w426) -> (element #1=w433:i32, element #2=w432:i32)  [unwired: 2 in]
                  n269 = for {
                    tunnel: w426 -> [w440]
                    tunnel: w427 -> [w439] mode=indexing
                    tunnel: [w438] -> w425
                    stop <- w438 stop-if-true
                    n270 = Equal?(x=w440, y=w439) -> (x = y?=w438:bool)
                  }
                  n271 = Index Array(array=w431, index=w433) -> (element=w430:string)
                  n272 = Index Array(array=w431, index=w432) -> (element=w429:string)
                  n273 = Format Into String(format string="%s & %s", w430, w429) -> (resulting string=w422:string)  [unwired: 2 in, 1 out]
                  n274 = case shown="True" w425 {
                    tunnel: w424 -> [w434 w437]
                    tunnel: [w434 w436] -> w423
                    tunnel: w422 -> [_ w435]
                    frame False {
                    }
                    frame True {
                      n275 = Build Array (concatenate)(w437, w435) -> (w436:string[])
                    }
                  }
                }
                n276 = case shown="\"Correlate without activating panel\"" w400 {
                  tunnel: w399 -> [_ w409 w413]
                  tunnel: w396 -> [_ w407 w414]
                  tunnel: w395 -> [_ w405 w415]
                  tunnel: [i32[][] [] ("Correlation Pairs") w403 w416] -> w394
                  frame "Cross correlation off" {
                  }
                  frame "Show correlation panel" {
                    n277 = call "Select_Strings.vi"("Available Ch names"=w409, "Message"="Please select Channels to Correlate", "Selector mode"=T14."Zero or more", "Desired Ch names (in)"=w407) -> ("Ch Indicies Choosen"=w404:i32[])  [unwired: 2 in, 2 out]
                    n278 = for {
                      tunnel: w405 -> [w412]
                      tunnel: w404 -> [w411] mode=indexing
                      tunnel: [w410] -> w403 mode=indexing
                      n279 = Index Array(array=w412, index (row)=w411) -> (element=w410:i32[])  [unwired: 1 in]
                    }
                  }
                  frame "Correlate without activating panel" {
                    n280 = for {
                      tunnel: [w421] -> w416 mode=indexing
                      tunnel: w415 -> [w420]
                      tunnel: w414 -> [w419] mode=indexing
                      tunnel: w413 -> [w418]
                      n281 = Search 1D Array(1D array=w418, element=w419) -> (index of element=w417:i32)  [unwired: 1 in]
                      n282 = Index Array(array=w420, index (row)=w417) -> (element=w421:i32[])  [unwired: 1 in]
                    }
                  }
                }
              }
              frame True {
              }
            }
          }
          frame #2 {
            n283 = for {
              shift-right: [w452] -> w442
              shift-left: i32[][] [] -> [w453]
              tunnel: w445 -> [w454]
              tunnel: w444 -> [w451] mode=indexing
              n284 = for {
                tunnel: w454 -> [w469] mode=indexing
                tunnel: w451 -> [w468]
                tunnel: [w467] -> w450
                stop <- w467 stop-if-true
                n285 = Equal?(x=w468, y=w469) -> (x = y?=w467:bool)
              }
              n286 = case shown="True" w450 {
                tunnel: w453 -> [w455 w457]
                tunnel: w451 -> [_ w458]
                tunnel: [w455 w459] -> w452
                frame False {
                }
                frame True {
                  n287 = for {
                    tunnel: w458 -> [w462]
                    tunnel: w457 -> [w461] mode=indexing
                    tunnel: [w460] -> w456
                    stop <- w460 stop-if-true
                    n288 = Equal?(x=w462, y=w461) -> (x = y?=w460:bool)
                  }
                  n289 = case shown="False" w456 {
                    tunnel: w457 -> [w465 w466]
                    tunnel: w458 -> [w464 _]
                    tunnel: [w463 w466] -> w459
                    frame False {
                      n290 = Build Array (concatenate)(w465, w464) -> (w463:i32[][])
                    }
                    frame True {
                    }
                  }
                }
              }
            }
            n291 = global write "Meas_global.vi" "correlate"(w442) -> ()
            n292 = Array Size(array=w442) -> (size(s)=w449:i32[])
            n293 = Index Array(array=w449, index=0) -> (element=w446:i32)
            n294 = Equal To 0?(x=w446) -> (x = 0?=w447:bool)
            n295 = case shown="True" w447 {
              frame False {
              }
              frame True {
                n296 = local write "Correlate?"(T9."Cross correlation off" ("Correlate?")) -> ()
              }
            }
          }
          frame #3 {
            n297 = Array Size(array=w474) -> (size(s)=w472:i32)
            n298 = Initialize Array(T15 {"Weighting"=[], "Time (ms)"=[], "Voltage"=[], "Eng Values"=[]} ("Time Trace"), w472) -> (w471:T29)
            n299 = global write "Meas_global.vi" "Time Trace"(w471) -> ()
          }
        }
      }
      frame #12 {
        n300 = stacked-sequence {
          seq-local: [w485 _] -> [_ w507]
          tunnel: w479 -> [w484 _]
          frame #0 {
            n301 = call "LDA+_An_Analysis_mode.vi"("Second Graph"="Second Graph", "First Graph"="First Graph") -> ("Second Graph out"=w480:T8, "First Graph out"=w482:T8)  [unwired: 6 out]
            n302 = case shown="False" w484 {
              tunnel: [w495 w506] -> w483
              tunnel: w482 -> [w494 w506]
              tunnel: [w493 w505] -> w481
              tunnel: w480 -> [w492 w505]
              frame False {
                w490 = Graph_Type."Show no graph" ("Plot Type")
                n303 = Unbundle By Name(w494) -> ("Save graph"=w496:u16)
                n304 = Unbundle By Name(w492) -> ("Save graph"=w491:u16)
                n305 = case shown="0, Default" w496 {
                  tunnel: [w502 w504] -> w495
                  tunnel: w494 -> [w503 w504]
                  tunnel: w490 -> [w501 _]
                  frame 0, Default {
                    n306 = Bundle By Name(cluster=w503, "Plot Type"=w501) -> (w502:T8)
                  }
                  frame 1 {
                  }
                }
                n307 = case shown="0, Default" w491 {
                  tunnel: [w498 w500] -> w493
                  tunnel: w492 -> [w499 w500]
                  tunnel: w490 -> [w497 _]
                  frame 0, Default {
                    n308 = Bundle By Name(cluster=w499, "Plot Type"=w497) -> (w498:T8)
                  }
                  frame 1 {
                  }
                }
              }
              frame True {
              }
            }
            n309 = local write "Second Graph"(w481) -> ()
            n310 = local write "First Graph"(w483) -> ()
            n311 = global write "Meas_global.vi" "Second Graph"(w481) -> ()
            n312 = global write "Meas_global.vi" "First Graph"(w483) -> ()
            n313 = Unbundle By Name(w481) -> ("Plot Type"=w489:T7)
            n314 = Unbundle By Name(w483) -> ("Plot Type"=w488:T7)
            n315 = Build Array(w488, w489) -> (w485:T7[])
          }
          frame #1 {
            n316 = global read "Meas_global.vi" "Insts for plotting"() -> (w508:u16[][])
            n317 = for {
              tunnel: w508 -> [w510] mode=indexing
              tunnel: w507 -> [w509] mode=indexing
              i -> [w511]
              n318 = stacked-sequence {
                seq-local: [w514 _] -> [_ w526]
                seq-local: [w515 _] -> [_ w525]
                tunnel: w511 -> [_ w529]
                tunnel: w510 -> [w513 _]
                tunnel: w509 -> [_ w521]
                frame #0 {
                  n319 = property on="Plot 1" class="Ring (strict)"() -> ("Strings []"=w512:string[])  [unwired: 2 in, 2 out]
                  n320 = Array To Cluster(array=w513) -> (cluster=w518:T30)
                  n321 = Unbundle(w518) -> ("Insts for plotting[0]"=w517:u16, "Insts for plotting[1]"=w516:u16)
                  n322 = Index Array(array=w512, index=w517) -> (element=w514:string)
                  n323 = Index Array(array=w512, index=w516) -> (element=w515:string)
                }
                frame #1 {
                  n324 = case shown="\"Show no graph\"" w521 {
                    tunnel: [u8 0 u8 0 u8 0 u8 0 u8 0 u8 1 u8 0] -> w533
                    tunnel: [u8 0 u8 0 u8 0 u8 0 u8 1 u8 1 u8 0] -> w532
                    tunnel: [u8 0 u8 0 u8 0 u8 0 u8 1 u8 1 u8 0] -> w531
                    tunnel: [u8 0 u8 0 u8 0 u8 0 u8 1 u8 0 u8 0] -> w530
                    tunnel: [FALSE TRUE TRUE TRUE TRUE TRUE TRUE] -> w524
                    tunnel: [u8 0 u8 1 u8 1 u8 2 u8 0 u8 0 u8 2] -> w523
                    tunnel: [u8 0 u8 4 u8 1 u8 2 u8 0 u8 0 u8 1] -> w522
                    tunnel: ["" "Time (s)" "Time (s)" "" "" "" ""] -> w520
                    tunnel: ["" "Voltage" "Velocity" "" "" "" ""] -> w519
                    frame "Show no graph" {
                    }
                    frame "Voltage trace" {
                    }
                    frame "Velocity trace" {
                    }
                    frame "Vel histogram" {
                    }
                    frame "Spectrum" {
                    }
                    frame "f.E(f) v Log f" {
                    }
                    frame "Auto-Corr" {
                    }
                  }
                  n325 = case shown="0, Default" w529 {
                    tunnel: w524 -> [w546 w559]
                    tunnel: w533 -> [w545 w558]
                    tunnel: w532 -> [w544 w557]
                    tunnel: w531 -> [w543 w556]
                    tunnel: w530 -> [w542 w555]
                    tunnel: u32 0 -> [w541 w554]
                    tunnel: u32 1 -> [w540 w552]
                    tunnel: w526 -> [w539 w553]
                    tunnel: w525 -> [w538 w551]
                    tunnel: w523 -> [w537 w550]
                    tunnel: w522 -> [w536 w549]
                    tunnel: w520 -> [w535 w548]
                    tunnel: w519 -> [w534 w547]
                    frame 0, Default {
                      n326 = property on="First plot" class="XYGraph (strict)"("Visible"=w546, "X Scale.Format & Precision:Format"=w545, "X Scale.Mapping Mode"=w544, "Y Scale.Format & Precision:Format"=w543, "Y Scale.Mapping Mode"=w542, "Active Plot"=w541, "Plot.Plot Name"=w539, "Active Plot"=w540, "Plot.Plot Name"=w538, "X Scale.Format & Precision:Precision"=w537, "Y Scale.Format & Precision:Precision"=w536, "XScale.NameLbl.Text"=w535, "YScale.NameLbl.Text"=w534) -> ()  [unwired: 2 in, 2 out]
                    }
                    frame 1 {
                      n327 = property on="2nd plot" class="XYGraph (strict)"("Visible"=w559, "X Scale.Format & Precision:Format"=w558, "X Scale.Mapping Mode"=w557, "Y Scale.Format & Precision:Format"=w556, "Y Scale.Mapping Mode"=w555, "Active Plot"=w554, "Plot.Plot Name"=w553, "Active Plot"=w552, "Plot.Plot Name"=w551, "X Scale.Format & Precision:Precision"=w550, "Y Scale.Format & Precision:Precision"=w549, "XScale.NameLbl.Text"=w548, "YScale.NameLbl.Text"=w547) -> ()  [unwired: 2 in, 2 out]
                    }
                  }
                }
              }
            }
          }
        }
      }
      frame #13 {
        n328 = local read "Second Graph"() -> (w634:T8)
        n329 = local read "First Graph"() -> (w633:T8)
        n330 = Unbundle By Name(w633) -> ("Plot 1"=w626:u16, "Plot 2"=w627:u16)
        n331 = Unbundle By Name(w634) -> ("Plot 1"=w628:u16, "Plot 2"=w629:u16)
        n332 = Build Array(w626, w627) -> (w630:u16[])
        n333 = Build Array(w628, w629) -> (w631:u16[])
        n334 = global read "Meas_global.vi" "Analysis Info cluster"() -> (w635:T22[])
        n335 = Decrement(x=w630) -> (x-1=w624:u16[])
        n336 = Decrement(x=w631) -> (x-1=w632:u16[])
        n337 = for {
          tunnel: w635 -> [w643]
          tunnel: w624 -> [w642] mode=indexing
          shift-right: [w636] -> _
          shift-left: u32 0 -> [w638]
          i -> [w637]
          n338 = Index Array(array=w643, index=w642) -> (element=w644:T22)
          n339 = Unbundle By Name(w644) -> ("Colour"=w639:u32)
          n340 = Equal?(x=w639, y=w638) -> (x = y?=w641:bool)
          n341 = Select(t=u32 13434624, s=w641, f=w639) -> (s? t:f=w636:u32)
          n342 = property on="First plot" class="XYGraph (strict)"("Active Plot"=w637, "Plot.Plot Color"=w636, "Plot.Fill/Point Color"=w636) -> ()  [unwired: 2 in, 2 out]
        }
        n343 = for {
          tunnel: w635 -> [w652]
          tunnel: w632 -> [w651] mode=indexing
          shift-right: [w647] -> _
          shift-left: u32 0 -> [w645]
          i -> [w650]
          n344 = Index Array(array=w652, index=w651) -> (element=w653:T22)
          n345 = Unbundle By Name(w653) -> ("Colour"=w646:u32)
          n346 = Equal?(x=w646, y=w645) -> (x = y?=w649:bool)
          n347 = Select(t=u32 13434624, s=w649, f=w646) -> (s? t:f=w647:u32)
          n348 = property on="2nd plot" class="XYGraph (strict)"("Active Plot"=w650, "Plot.Plot Color"=w647, "Plot.Fill/Point Color"=w647) -> ()  [unwired: 2 in, 2 out]
        }
      }
      frame #14 {
        n349 = global read "DataTranslation_global.vi" "Different Sampling Freq per block"() -> (w654:bool)
        n350 = global read "Meas_global.vi" "Remote control"() -> (w663:bool)
        n351 = global read "Meas_global.vi" "Post Process"() -> (w666:T2)
        n352 = global read "Meas_global.vi" "PWA Data"() -> (w655:T31)
        n353 = case shown="\"No PWA Data\"" w655 {
          tunnel: [w674 w679] -> w657
          frame "No PWA Data" {
            n354 = local read "Desired Sampling freq (Hz)"() -> (w676:dbl)
            n355 = local read "No of samples"() -> (w675:i32)
            n356 = Divide(x=w675, y=w676) -> (x/y=w674:dbl)
          }
          frame "One Ch PWA" {
            n357 = local read "No of samples"() -> (w677:i32)
            n358 = global read "PWAtasksGLOBAL.vi" "PWA Freq. (Hz)"() -> (w678:dbl)
            n359 = global write "PWAtasksGLOBAL.vi" "PWA No. of Samples"(w677) -> ()
            n360 = Divide(x=w677, y=w678) -> (x/y=w679:dbl)
          }
        }
        n361 = Equal?(x=Setup."Run Program" ("setup"), y=w660) -> (x = y?=w658:bool)
        n362 = global read "Meas_global.vi" "Averaging time (min)"() -> (w661:dbl)
        n363 = Equal?(x=Post_Process."Take New Data" ("Post Process"), y=w666) -> (x = y?=w662:bool)
        n364 = Compound Arithmetic op=AND(invert w654, w662, invert w656, invert w663, w658) -> (w664:bool)
        n365 = case shown="True" w664 {
          tunnel: w661 -> [_ w673]
          tunnel: w657 -> [_ w672]
          frame False {
          }
          frame True {
            n366 = Multiply(x=w673, y=60.0) -> (x*y=w669:dbl)
            n367 = Divide(x=w669, y=w672) -> (x/y=w668:dbl)
            n368 = Round Toward +Infinity(x=w668) -> (ceil(x): smallest int >= x=w667:dbl)
            n369 = To Long Integer(number=w667) -> (32bit integer=w671:i32)
            n370 = global write "Meas_global.vi" "Requested No of blocks"(w671) -> ()
            n371 = local write "No of Blocks"(w671) -> ()
          }
        }
      }
      frame #15 {
        n372 = case shown="\"Run Program\"" w680 {
          frame "Run Program" {
            n373 = call "Read_calibration_files.vi"() -> ()  [unwired: 1 out]
            n374 = global write "Meas_global.vi" "Repeat Measurement?"(FALSE ("Repeat Measurement?")) -> ()
          }
          frame "Show Setup", Default {
          }
        }
      }
      frame #16 {
        n375 = global read "Meas_global.vi" "Raw data option"() -> (w685:enum16{"Save raw data", "Raw data not saved"})
        n376 = Get Date/Time In Seconds() -> (seconds since 1Jan1904=w686:timestamp)
        n377 = To Double Precision Float(number=w686) -> (double precision float=w683:dbl)
        n378 = global read "Meas_global.vi" "Post Process"() -> (w684:T2)
        n379 = case shown="\"Setup Front Panel\"" w687 {
          tunnel: w685 -> [w689 _ _ _]
          tunnel: w684 -> [w688 _ w730 w739]
          frame "Run Program" {
            n380 = case shown="\"Take New Data\"" w688 {
              tunnel: w689 -> [w699 _]
              frame "Take New Data" {
                n381 = case shown="\"Save raw data\"" w699 {
                  frame "Save raw data" {
                  }
                  frame "Raw data not saved" {
                    w707 = FALSE  # Lock File
                    w704 = FALSE  # advisory dialog? (display:T)
                    w703 = FALSE  # append to file? (new file:F)
                    n382 = global read "Meas_global.vi" "Remote control"() -> (w705:bool)
                    n383 = call "Create_setup_string.vi"() -> ("Setup String"=w708:string)  [unwired: 1 out]
                    n384 = case shown="False" w705 {
                      tunnel: ["Current_Setup.xls" ("Setup filename") w710] -> w700
                      frame False {
                      }
                      frame True {
                        n385 = local read "Setup filename"() -> (w710:string)
                      }
                    }
                    n386 = call "Add_length_to_string.vi"("String in"=w708) -> ("String out"=w706:string)
                    n387 = call "Setup_Filepath.vi"("Setup File Type"=Setup_Filetype."Measurement Setups", "Filename in"=w700) -> ("Filename Out"=w701:path)  [unwired: 1 out]
                    n388 = call "Write_Characters_To_File.vi"("file path (dialog if empty)"=w701, "advisory dialog? (display:T)"=w704, "character string"=w706, "append to file? (new file:F)"=w703, "Lock File"=w707) -> ()  [unwired: 4 out]
                  }
                }
                n389 = global read "Meas_global.vi" "Requested No of samples"() -> (w693:i32)
                n390 = global read "Meas_global.vi" "Requested Sampling rate"() -> (w696:dbl)
                n391 = global read "Meas_global.vi" "Requested No of blocks"() -> (w692:i32)
                n392 = Divide(x=w693, y=w696) -> (x/y=w695:dbl)
                n393 = Multiply(x=w692, y=w695) -> (x*y=w691:dbl)
                n394 = Add(x=w691, y=120.0) -> (x+y=w690:dbl)
                n395 = call "Program_Active_Client.vi"("Mode"=enum16{"Program Active", "Traverse Level State"}."Program Active", "Time till next contact (Sec)"=w690, "Traverse level State"=Traverse_Level_State."Running") -> ()  [unwired: 3 out]
              }
              frame "Post Process Raw Data File" {
              }
            }
          }
          frame "Save Current Setup" {
            n396 = stacked-sequence {
              seq-local: [w713 _] -> [_ w716]
              seq-local: [w712 _] -> [_ w715]
              frame #0 {
                w714 = FALSE  # Save New File?
                n397 = call "Save_current_setup.vi"("Save New File?"=w714, "Setup File Type"=Setup_Filetype."Measurement Setups") -> ("Cancelled?"=w712:bool, "Saved filepath"=w713:path)  [unwired: 2 out]
              }
              frame #1 {
                n398 = case shown="False" w715 {
                  tunnel: w716 -> [w722 _]
                  frame False {
                    w719 = "Initial Probe positions" ("File Label")
                    w727 = FALSE  # append to file? (new file:F)
                    w728 = FALSE  # advisory dialog? (display:T)
                    w729 = FALSE  # Lock File
                    n399 = call "Input_Instrument_Positions.vi"("Filepath to Save"=w722) -> ("Output string"=w721:string)  [unwired: 1 out]
                    n400 = call "Create_setup_string.vi"() -> ("Setup String"=w720:string)  [unwired: 1 out]
                    n401 = call "Get_string_subset.vi"("String to split"=w721, "File Label"=w719) -> ("Output string"=w718:string)  [unwired: 2 in, 1 out]
                    n402 = call "Replace_data_in_Label_str.vi"("New data string"=w718, "Input string"=w720, "Variable name"=w719) -> ("Appended string"=w717:string)
                    n403 = call "Replace_data_in_setup_string.vi"("New data string"="", "Input string"=w717, "Variable name"="Comments") -> ("Appended string"=w723:string)
                    n404 = call "Add_length_to_string.vi"("String in"=w723) -> ("String out"=w726:string)
                    n405 = call "Write_Characters_To_File.vi"("file path (dialog if empty)"=w722, "advisory dialog? (display:T)"=w728, "character string"=w726, "append to file? (new file:F)"=w727, "Lock File"=w729) -> ()  [unwired: 4 out]
                  }
                  frame True {
                  }
                }
              }
            }
          }
          frame "Show Setup" {
            n406 = case shown="\"Take New Data\"" w730 {
              frame "Take New Data" {
                w735 = FALSE  # append to file? (new file:F)
                w736 = FALSE  # advisory dialog? (display:T)
                w737 = FALSE  # Lock File
                n407 = call "Create_setup_string.vi"() -> ("Setup String"=w738:string)  [unwired: 1 out]
                n408 = call "Add_length_to_string.vi"("String in"=w738) -> ("String out"=w734:string)
                n409 = call "Setup_Filepath.vi"("Setup File Type"=Setup_Filetype."Measurement Setups", "Filename in"="Current_Setup.xls" ("Setup filename")) -> ("Filename Out"=w732:path)  [unwired: 1 out]
                n410 = call "Write_Characters_To_File.vi"("file path (dialog if empty)"=w732, "advisory dialog? (display:T)"=w736, "character string"=w734, "append to file? (new file:F)"=w735, "Lock File"=w737) -> ()  [unwired: 4 out]
              }
              frame "Post Process Raw Data File" {
              }
            }
          }
          frame "Setup Front Panel" {
            n411 = case shown="\"Take New Data\"" w739 {
              frame "Take New Data" {
                w744 = FALSE  # append to file? (new file:F)
                w745 = FALSE  # advisory dialog? (display:T)
                w746 = FALSE  # Lock File
                n412 = call "Create_setup_string.vi"() -> ("Setup String"=w747:string)  [unwired: 1 out]
                n413 = call "Add_length_to_string.vi"("String in"=w747) -> ("String out"=w743:string)
                n414 = call "Setup_Filepath.vi"("Setup File Type"=Setup_Filetype."Measurement Setups", "Filename in"="Current_Setup.xls" ("Setup filename")) -> ("Filename Out"=w741:path)  [unwired: 1 out]
                n415 = call "Write_Characters_To_File.vi"("file path (dialog if empty)"=w741, "advisory dialog? (display:T)"=w745, "character string"=w743, "append to file? (new file:F)"=w744, "Lock File"=w746) -> ()  [unwired: 4 out]
              }
              frame "Post Process Raw Data File" {
              }
            }
          }
        }
        n416 = global write "Meas_global.vi" "Actual Measurement time (min)"(0.0 ("Max Measurement time (min)")) -> ()
      }
      frame #17 {
        n417 = case shown="\"Setup Front Panel\", Default" w751 {
          tunnel: w748 -> [w753 _]
          tunnel: w750 -> [_ w846]
          tunnel: w749 -> [w752 _]
          frame "Run Program" {
            n418 = while {
              tunnel: w753 -> [w755]
              tunnel: w752 -> [w754]
              i -> [w756]
              stop <- w757 stop-if-true
              n419 = Increment(x=w756) -> (x+1=w758:i32)
              n420 = stacked-sequence {
                seq-local: [_ _ _ _ _ "Block average display control" _ _ _ _] -> [_ _ _ _ _ _ w791 _ _ _]
                seq-local: [_ _ _ _ _ _ w789 _ _ _] -> [_ _ _ _ _ _ _ w807 _ _]
                seq-local: [_ _ _ _ w772 _ _ _ _ _] -> [_ _ _ _ _ _ _ _ _ w839]
                seq-local: [_ w760 _ _ _ _ _ _ _ _] -> [_ _ w764 _ _ _ _ _ _ _]
                seq-local: [_ _ w762 _ _ _ _ _ _ _] -> [_ _ _ _ _ _ _ _ _ w842]
                tunnel: w758 -> [w759 _ w763 _ _ w781 _ _ _ w843]
                tunnel: [_ _ w762 _ _ _ _ _ _ _] -> w757
                tunnel: w755 -> [_ _ _ _ w771 _ _ _ _ _]
                tunnel: w754 -> [_ _ _ _ _ _ _ _ _ _]
                frame #0 {
                  n421 = global write "Meas_global.vi" "Current Block No"(w759) -> ()
                  "Current Block No" <- w759
                }
                frame #1 {
                  n422 = call "Get_data.vi"() -> ("EOF? and Error status"=w760:bool, "Block Header"=w761:string)  [unwired: 10 out]
                  n423 = global write "Plug_in_data_global.vi" "Block Header"(w761) -> ()
                }
                frame #2 {
                  w766 = string[] [] ("Plug in titles")
                  n424 = global write "Meas_global.vi" "Requested No of blocks"("No of Blocks") -> ()
                  n425 = Less Or Equal?(x="No of Blocks", y=w763) -> (x <= y?=w767:bool)
                  n426 = Compound Arithmetic op=OR(w764, w767) -> (w762:bool)
                  n427 = case shown="True" w762 {
                    tunnel: w763 -> [_ w768]
                    frame False {
                    }
                    frame True {
                      n428 = global write "Meas_global.vi" "Requested No of blocks"(w768) -> ()
                      n429 = local write "No of Blocks"(w768) -> ()
                    }
                  }
                  n430 = global write "Meas_global.vi" "Processing last block?"(w762) -> ()
                  n431 = global write "Dynamic_call_global.ph.vi" "Plug in values"(w766) -> ()
                  n432 = global write "Dynamic_call_global.ph.vi" "Plug in titles"(w766) -> ()
                  n433 = global write "PWAtasksGLOBAL.vi" "STOP"(w762) -> ()
                }
                frame #3 {
                  n434 = call "Text_without_format.vi"("Input string"="Comments") -> ("Output string"=w769:string)
                  n435 = local write "Comments"(w769) -> ()
                  n436 = global write "Meas_global.vi" "Comments"(w769) -> ()
                }
                frame #4 {
                  n437 = call "Process_data.vi"("Measurement top level?"=w771) -> ("Vel stat display"=→"Statistics":string[][], "First Plot data Cluster"=→"First plot":cluster{"X array":dbl[], "Y array":dbl[]}[], "Second Plot Data Cluster"=→"2nd plot":cluster{"X array":dbl[], "Y array":dbl[]}[], "Max Measurement time up"=w772:bool)  [unwired: 5 in]
                }
                frame #5 {
                  n438 = global read "Meas_global.vi" "Actual Measurement time (min)"() -> (→"Measurement time (min)":dbl)
                  n439 = global read "Meas_global.vi" "Actual Sampling rate (Hz)"() -> (→"Actual Sampling freq":dbl)
                  n440 = call "Display_blocks.vi"("Block No"=w781, "Block average display"="Block average display control") -> ("u^4"=→"u^4":dbl[][], "u^3"=→"u^3":dbl[][], "uv"=→"uv":dbl[][], "u^2"=→"u^2" →"Array u^2":dbl[][], "U"=→"U" →"Array U":dbl[][])  [unwired: 4 out]
                }
                frame #6 {
                  n441 = global read "Meas_global.vi" "Analysis Info cluster"() -> (w790:T22[])
                  n442 = global read "Meas_global.vi" "Diagnostic info"() -> (w788:string[][])
                  n443 = for {
                    tunnel: w791 -> [w806] mode=indexing
                    tunnel: w790 -> [w803] mode=indexing
                    tunnel: [w805] -> w789 mode=indexing if=w804
                    tunnel: [w793] -> w787 mode=indexing
                    tunnel: [w792] -> w786 mode=indexing
                    n444 = Unbundle By Name(w803) -> ("Colour"=w805:u32)
                    n445 = Unbundle By Name(w806) -> ("Include"=w804:bool)
                    n446 = Unbundle By Name(w803) -> ("Inst name"=w797:string, "Av Sampling Rate"=w799:dbl, "Av No of Samples"=w796:dbl)
                    n447 = Format Into String(format string="%s Freq Hz", w797) -> (resulting string=w801:string)  [unwired: 2 in, 1 out]
                    n448 = Format Into String(format string="%s Samples per block", w797) -> (resulting string=w794:string)  [unwired: 2 in, 1 out]
                    n449 = Number To Decimal String(number=w799) -> (decimal integer string=w800:string)  [unwired: 1 in]
                    n450 = Number To Decimal String(number=w796) -> (decimal integer string=w795:string)  [unwired: 1 in]
                    n451 = Build Array(w801, w800) -> (w793:string[])
                    n452 = Build Array(w794, w795) -> (w792:string[])
                  }
                  n453 = Build Array (concatenate)(w788, w787, w786) -> (→"Diagnostic info":string[][])
                }
                frame #7 {
                  n454 = for {
                    tunnel: w807 -> [w808] mode=indexing
                    i -> [w809]
                    n455 = property on="U" class="WFGraph (strict)"("Active Plot"=w809, "Plot.Plot Color"=w808, "Plot.Fill/Point Color"=w808) -> ()  [unwired: 2 in, 2 out]
                    n456 = property on="u^3" class="WFGraph (strict)"("Active Plot"=w809, "Plot.Plot Color"=w808, "Plot.Fill/Point Color"=w808) -> ()  [unwired: 2 in, 2 out]
                    n457 = property on="u^4" class="WFGraph (strict)"("Active Plot"=w809, "Plot.Plot Color"=w808, "Plot.Fill/Point Color"=w808) -> ()  [unwired: 2 in, 2 out]
                    n458 = property on="u^2" class="WFGraph (strict)"("Active Plot"=w809, "Plot.Plot Color"=w808, "Plot.Fill/Point Color"=w808) -> ()  [unwired: 2 in, 2 out]
                  }
                }
                frame #8 {
                  n459 = case shown="True" "Pause" {
                    frame False {
                    }
                    frame True {
                      n460 = global read "Meas_global.vi" "Post Process"() -> (w811:T2)
                      n461 = case shown="\"Take New Data\"" w811 {
                        frame "Take New Data" {
                          n462 = call "Program_Active_Client.vi"("Mode"=enum16{"Program Active", "Traverse Level State"}."Program Active", "Time till next contact (Sec)"=12000.0, "Traverse level State"=Traverse_Level_State."Running") -> ()  [unwired: 3 out]
                          n463 = while {
                            i -> [w818]
                            stop <- w819 continue-if-true
                            n464 = Quotient & Remainder(x=w818, y=10) -> (x-y*floor(x/y)=w816:i32)  [unwired: 1 out]
                            n465 = Equal To 0?(x=w816) -> (x = 0?=w815:bool)
                            n466 = stacked-sequence {
                              seq-local: [_ w821 _ _] -> [_ _ w823 _]
                              tunnel: [_ w821 _ _] -> w819
                              tunnel: w815 -> [_ _ _ w825]
                              frame #0 {
                                "Pause message" <- "Measurement Program Paused!!!!" ("Pause message")
                              }
                              frame #1 {
                                n467 = global write "Trav_pos_global.vi" "Paused During Row?"(TRUE ("Paused During Row?")) -> ()
                                n468 = local read "Pause"() -> (w821:bool)
                              }
                              frame #2 {
                                n469 = property on="Pause message" class="Str"("Blinking"=w823, "Visible"=w823) -> ()  [unwired: 2 in, 2 out]
                                n470 = Wait Until Next ms Multiple(millisecond multiple=u32 1000) -> ()  [unwired: 1 out]
                              }
                              frame #3 {
                                n471 = case shown="False" w825 {
                                frame False {
                                }
                                frame True {
                                n472 = Current VI's Path() -> (path=w826:path)
                                n473 = call "Bring_to_front.vi"("path"=w826) -> ()
                                }
                                }
                              }
                            }
                          }
                        }
                        frame "Post Process Raw Data File" {
                          n474 = stacked-sequence {
                            seq-local: [_ w829 _ _] -> [_ _ _ w836]
                            frame #0 {
                              n475 = property on="PP next block" class="Bool (strict)"("Visible"=TRUE) -> ()  [unwired: 2 in, 2 out]
                              n476 = local write "PP next block"(FALSE ("PP next block")) -> ()
                            }
                            frame #1 {
                              n477 = while {
                                tunnel: [w833] -> w829
                                stop <- w830 stop-if-true
                                n478 = local read "stop"() -> (w833:bool)
                                n479 = local read "Pause"() -> (w831:bool)
                                n480 = Compound Arithmetic op=OR(w833, "PP next block", invert w831) -> (w830:bool)
                                n481 = case shown="False" w830 {
                                frame False {
                                n482 = Wait (ms)(milliseconds to wait=u32 200) -> ()  [unwired: 1 out]
                                }
                                frame True {
                                }
                                }
                              }
                            }
                            frame #2 {
                              n483 = property on="PP next block" class="Bool (strict)"("Visible"=FALSE) -> ()  [unwired: 2 in, 2 out]
                            }
                            frame #3 {
                              n484 = Stop(stop? (T)=w836) -> ()
                            }
                          }
                        }
                      }
                    }
                  }
                }
                frame #9 {
                  n485 = global read "Meas_global.vi" "stop"() -> (w837:bool)
                  n486 = Compound Arithmetic op=OR("stop", w839, w837) -> (w838:bool)
                  n487 = Compound Arithmetic op=AND(w838, invert w842) -> (w841:bool)
                  n488 = case shown="True" w841 {
                    tunnel: w843 -> [_ w845]
                    frame False {
                    }
                    frame True {
                      n489 = Increment(x=w845) -> (x+1=w844:i32)
                      n490 = local write "No of Blocks"(w844) -> ()
                      n491 = global write "Meas_global.vi" "Requested No of blocks"(w844) -> ()
                    }
                  }
                }
              }
            }
          }
          frame "Setup Front Panel", Default {
            n492 = stacked-sequence {
              seq-local: [w847 _ _ _ _ _ _] -> [_ _ _ _ _ w927 _]
              seq-local: [_ w853 _ _ _ _ _] -> [_ _ _ _ _ w926 _]
              seq-local: [_ _ _ w885 _ _ _] -> [_ _ _ _ _ w925 _]
              seq-local: [_ _ _ _ w903 _ _] -> [_ _ _ _ _ w923 _]
              seq-local: [_ w852 _ _ _ _ _] -> [_ _ _ _ _ _ w936]
              seq-local: [_ _ w878 _ _ _ _] -> [_ _ _ _ _ w922 _]
              tunnel: w846 -> [_ w854 _ _ _ _ _]
              frame #0 {
                n493 = Build Array("Name", "Channel", "High limit", "Low limit") -> (w847:string[])
              }
              frame #1 {
                n494 = global read "Meas_global.vi" "LDA data"() -> (w852:enum16{"No LDA data", "Take LDA data"})
                n495 = case shown="\"Take LDA data\"" w852 {
                  tunnel: w854 -> [_ w865]
                  tunnel: [string[][] [] w862] -> w853
                  frame "No LDA data" {
                  }
                  frame "Take LDA data" {
                    n496 = global read "LDA_meas_global_1.vi" "Max Vel BSA1"() -> (w857:dbl)
                    n497 = global read "LDA_meas_global_1.vi" "Min Vel BSA1"() -> (w856:dbl)
                    n498 = global read "LDA_meas_global_1.vi" "Vel Comp BSA1"() -> (w866:string)
                    n499 = case shown="\"2D\"" w865 {
                      tunnel: [string[] [] w871] -> w863
                      frame "1D" {
                      }
                      frame "2D" {
                        n500 = global read "LDA_meas_global_2.vi" "Max Vel BSA2"() -> (w870:dbl)
                        n501 = global read "LDA_meas_global_2.vi" "Min Vel BSA2"() -> (w869:dbl)
                        n502 = global read "LDA_meas_global_2.vi" "Vel Comp BSA2"() -> (w872:string)
                        n503 = Format Into String(format string="%.1f m/s" ("Format String"), w869) -> (resulting string=w877:string)  [unwired: 2 in, 1 out]
                        n504 = Format Into String(format string="%.1f m/s" ("Format String"), w870) -> (resulting string=w876:string)  [unwired: 2 in, 1 out]
                        n505 = Build Array("LDA", w872, w876, w877) -> (w871:string[])
                      }
                    }
                    n506 = Format Into String(format string="%.1f m/s" ("Format String"), w856) -> (resulting string=w858:string)  [unwired: 2 in, 1 out]
                    n507 = Format Into String(format string="%.1f m/s" ("Format String"), w857) -> (resulting string=w859:string)  [unwired: 2 in, 1 out]
                    n508 = Build Array("LDA", w866, w859, w858) -> (w864:string[])
                    n509 = Build Array(w864, w863) -> (w862:string[][])
                  }
                }
              }
              frame #2 {
                n510 = global read "Meas_global.vi" "PWA Data"() -> (w879:T31)
                n511 = case shown="\"One Ch PWA\"" w879 {
                  tunnel: [string[][] [] w881] -> w878
                  frame "No PWA Data" {
                  }
                  frame "One Ch PWA" {
                    n512 = Build Array("PWA") -> (w882:string[])
                    n513 = Build Array(w882) -> (w881:string[][])
                  }
                }
              }
              frame #3 {
                n514 = global read "Meas_global.vi" "Acquisition vi to Run"() -> (w884:string)
                n515 = global read "Meas_global.vi" "Ch & spans"() -> (w886:T28[])
                n516 = for {
                  tunnel: w886 -> [w890] mode=indexing
                  tunnel: [w902] -> w885 mode=indexing
                  tunnel: w884 -> [w888]
                  n517 = Unbundle By Name(w890) -> ("DAQmx Chan"=w895:tag, "Var name"=w894:string, "Ch No"=w893:i16, "high limit (10V)"=w892:sgl, "low limit (-10V)"=w891:sgl)
                  n518 = Equal?(x=w888, y="NI-DAQmx.vi") -> (x = y?=w889:bool)
                  n519 = Number To Decimal String(number=w893) -> (decimal integer string=w896:string)  [unwired: 1 out]
                  n520 = Format Into String(format string="%.1f Volts" ("Format String"), w892) -> (resulting string=w899:string)  [unwired: 2 in, 1 out]
                  n521 = Format Into String(format string="%.1f Volts" ("Format String"), w891) -> (resulting string=w898:string)  [unwired: 2 in, 1 out]
                  n522 = Select(t=w895, s=w889, f=w896) -> (s? t:f=w897:string)
                  n523 = Build Array(w894, w897, w899, w898) -> (w902:string[])
                }
              }
              frame #4 {
                n524 = global read "Meas_global.vi" "Analysis Info cluster"() -> (w911:T22[])
                n525 = for {
                  tunnel: w911 -> [w921] mode=indexing
                  tunnel: [w920] -> w909 mode=indexing
                  n526 = Unbundle By Name(w921) -> ("Inst name"=w920:string)
                }
                n527 = global read "Meas_global.vi" "correlate"() -> (w910:i32[][])
                n528 = for {
                  tunnel: w910 -> [w916] mode=indexing
                  tunnel: w909 -> [w915]
                  tunnel: "Correlating" -> [w914]
                  tunnel: [w912] -> w904 mode=indexing
                  n529 = for {
                    tunnel: w916 -> [w919] mode=indexing
                    tunnel: w915 -> [w918]
                    tunnel: [w917] -> w913 mode=indexing
                    n530 = Index Array(array=w918, index=w919) -> (element=w917:string)
                  }
                  n531 = Build Array (concatenate)(w914, w913) -> (w912:string[])
                }
                n532 = Initialize Array("", 5 ("Dimension Size")) -> (w905:string[])
                n533 = Build Array (concatenate)(w905, w904) -> (w903:string[][])
              }
              frame #5 {
                n534 = Build Array (concatenate)(w927, w926, w922, w925, w923) -> (w924:string[][])
                n535 = local write "Statistics"(w924) -> ()
              }
              frame #6 {
                n536 = case shown="\"Take LDA data\"" w936 {
                  tunnel: [string[] [] w938] -> w933
                  frame "No LDA data" {
                  }
                  frame "Take LDA data" {
                    n537 = global read "Meas_global.vi" "Synchronise with LDA"() -> (w943:bool)
                    n538 = global read "Meas_global.vi" "Ch & spans"() -> (w946:T28[])
                    n539 = Array Size(array=w946) -> (size(s)=w945:i32)
                    n540 = Greater Than 0?(x=w945) -> (x > 0?=w944:bool)
                    n541 = Compound Arithmetic op=AND(w943, w944) -> (w942:bool)
                    n542 = Select(t="Synchronised with LDA", s=w942, f="") -> (s? t:f=w939:string)
                    n543 = Build Array(w939) -> (w938:string[])
                  }
                }
                n544 = global read "Meas_global.vi" "Continuous time trace?"() -> (w928:bool)
                n545 = Select(t="Continuous Time Trace", s=w928, f="") -> (s? t:f=w932:string)
                n546 = Build Array (concatenate)(w933, w932) -> (w931:string[])
                n547 = Build Array(w931) -> (w930:string[][])
                n548 = Transpose 2D Array(2D array=w930) -> (transposed array=w929:string[][])
                n549 = local write "Diagnostic info"(w929) -> ()
              }
            }
          }
        }
      }
      frame #18 {
        n550 = local read "File"() -> (w957:T5)
        n551 = Equal?(x=Setup."Run Program" ("setup"), y=w958) -> (x = y?=w955:bool)
        n552 = Not Equal?(x=w957, y=Save_Data."Save No Data" ("File")) -> (x != y?=w956:bool)
        n553 = global read "Meas_global.vi" "Repeat Measurement?"() -> (w947:bool)
        n554 = Compound Arithmetic op=AND(invert w947, w955, w956) -> (w954:bool)
        n555 = Get Date/Time In Seconds() -> (seconds since 1Jan1904=w951:timestamp)
        n556 = To Double Precision Float(number=w951) -> (double precision float=w949:dbl)
        n557 = local read "Setup filename"() -> (w952:string)
        n558 = case shown="True" w954 {
          tunnel: w957 -> [_ _]
          tunnel: w949 -> [w961 w994]
          tunnel: w952 -> [w960 w993]
          tunnel: w948 -> [w959 w992]
          frame True {
            n559 = stacked-sequence {
              seq-local: [_ w965 _] -> [_ _ w985]
              tunnel: w961 -> [w964 _ _]
              tunnel: w960 -> [w963 _ _]
              tunnel: w959 -> [w962 _ _]
              frame #0 {
                n560 = call "Write_Results_file.vi"("Experiment start time"=w962, "Experiment End time"=w964, "Setup filename"=w963) -> ()  [unwired: 4 out]
              }
              frame #1 {
                w970 = FALSE  # Empty list
                n561 = global read "Meas_global.vi" "Raw data file"() -> (w969:path)
                n562 = global read "Trav_pos_global.vi" "Top level setup filename"() -> (w967:path)
                n563 = global read "Meas_global.vi" "Start Time of experiment"() -> (w966:dbl)
                n564 = Strip Path(path=w969) -> (stripped path=w965:path)  [unwired: 1 out]
                n565 = Empty String/Path?(string/path=w967) -> (empty?=w968:bool)
                n566 = case shown="False" w968 {
                  tunnel: w967 -> [w984 _]
                  tunnel: w965 -> [w982 _]
                  tunnel: w966 -> [w980 _]
                  frame False {
                    n567 = call "Sec_to_date_filename.vi"("seconds"=w980) -> ("Day"=w979:string, "Time"=w978:string)  [unwired: 2 out]
                    n568 = Format Into String(format string="Cmd_%s_%s.xls", w979, w978) -> (resulting string=w976:string)  [unwired: 2 in, 1 out]
                    n569 = call "Fast_string_Replace.vi"("Replace match with:"="-", "Input String"=w976, "regular expression"=":") -> ("Output String"=w973:string)  [unwired: 2 out]
                    n570 = call "Fast_string_Replace.vi"("Replace match with:"="", "Input String"=w973, "regular expression"=" ") -> ("Output String"=w971:string)  [unwired: 2 out]
                    n571 = Build Path(base path=w982, name or relative path=w971) -> (appended path=w981:path)
                    n572 = Copy(10:w981, 11:w984) -> ()  [unwired: 1 in, 5 out]
                  }
                  frame True {
                  }
                }
                n573 = call "Remember_RD_Folders.vi"("Empty list"=w970, "Folders to Remember"=w965) -> ()  [unwired: 1 out]
              }
              frame #2 {
                n574 = global read "Meas_global.vi" "LDA data"() -> (w986:enum16{"No LDA data", "Take LDA data"})
                n575 = case shown="\"Take LDA data\"" w986 {
                  tunnel: w985 -> [_ w990]
                  frame "No LDA data" {
                  }
                  frame "Take LDA data" {
                    w988 = "LDA_Probe_Orientation.txt" ("name or relative path")
                    n576 = call "Setup_Filepath.vi"("Setup File Type"=Setup_Filetype."General", "Filename in"=w988) -> ("Filename Out"=w987:path)  [unwired: 1 out]
                    n577 = Build Path(base path=w990, name or relative path=w988) -> (appended path=w991:path)
                    n578 = Copy(10:w991, 11:w987) -> ()  [unwired: 1 in, 5 out]
                  }
                }
              }
            }
          }
          frame False {
            n579 = global read "Meas_global.vi" "Raw data option"() -> (w995:enum16{"Save raw data", "Raw data not saved"})
            n580 = case shown="\"Save raw data\"" w995 {
              tunnel: w992 -> [w998 _]
              tunnel: w994 -> [w997 _]
              tunnel: w993 -> [w996 _]
              frame "Save raw data" {
                n581 = stacked-sequence {
                  tunnel: w998 -> [_ w1007]
                  tunnel: w997 -> [_ w1006]
                  tunnel: w996 -> [_ w1004]
                  frame #0 {
                    n582 = global read "Meas_global.vi" "Current Block No"() -> (w999:i32)
                    n583 = global write "Meas_global.vi" "Requested No of blocks"(w999) -> ()
                  }
                  frame #1 {
                    n584 = call "Create_Raw_data_file.vi"("No of averages"=1, "End time"=w1006, "Start time"=w1007, "Setup filename"=w1004) -> ("Values"=w1002:string[][], "Column headers"=w1003:string[])  [unwired: 2 out]
                    n585 = Index Array(array=w1002, index (row)=0) -> (element=w1000:string[])  [unwired: 1 in]
                    n586 = global write "Dynamic_call_global.ph.vi" "Plug in values"(w1000) -> ()
                    n587 = global write "Dynamic_call_global.ph.vi" "Plug in titles"(w1003) -> ()
                  }
                }
              }
              frame "Raw data not saved" {
              }
            }
          }
        }
      }
      frame #19 {
        n588 = stacked-sequence {
          seq-local: [w1014 _] -> [_ w1023]
          seq-local: [w1010 _] -> [_ w1022]
          tunnel: w1008 -> [w1021 _]
          frame #0 {
            n589 = global read "Meas_global.vi" "Raw data file"() -> (w1012:path)
            n590 = global read "Meas_global.vi" "Raw data option"() -> (w1020:enum16{"Save raw data", "Raw data not saved"})
            n591 = Equal?(x=Setup."Run Program" ("setup"), y=w1021) -> (x = y?=w1016:bool)
            n592 = Strip Path(path=w1012) -> (stripped path=w1011:path)  [unwired: 1 out]
            n593 = Equal?(x=w1020, y=enum16{"Save raw data", "Raw data not saved"}."Save raw data" ("Raw data option")) -> (x = y?=w1015:bool)
            n594 = Build Path(base path=w1011, name or relative path="VI_History.xls") -> (appended path=w1010:path)
            n595 = call "Does_file_exist_(simple).vi"("Pathname"=w1010) -> ("exists?"=w1018:bool)
            n596 = Not(x=w1018) -> (.not. x?=w1017:bool)
            n597 = Compound Arithmetic op=AND(w1017, w1016, w1015) -> (w1014:bool)
          }
          frame #1 {
            n598 = case shown="True" w1023 {
              tunnel: w1022 -> [_ w1024]
              frame False {
              }
              frame True {
                n599 = stacked-sequence {
                  tunnel: w1024 -> [w1030 w1038]
                  frame #0 {
                    w1027 = FALSE  # Lock File
                    n600 = global read "Meas_global.vi" "ProgRevisionInfo"() -> (w1026:string)
                    n601 = call "Characters_to_string.vi"("Characters to write"=w1026, "Label for characters"="Prog Revision info") -> ("Output string"=w1032:string)
                    n602 = call "Date_and_Time_to_string.vi"() -> ("Date and time (spreadsheet)"=w1033:string)
                    n603 = call "Get_mod_dates.vi"() -> ("error out"=w1031:errorcluster, "Output string"=w1028:string)  [unwired: 1 in, 3 out]
                    n604 = call "EnFlo_Error_Handler.vi"("error in (no error)"=w1031) -> ()  [unwired: 2 in, 3 out]
                    n605 = Concatenate Strings(w1033, w1032, w1028) -> (w1029:string)
                    n606 = call "Write_Characters_To_File.vi"("file path (dialog if empty)"=w1030, "character string"=w1029, "Lock File"=w1027) -> ()  [unwired: 2 in, 4 out]
                  }
                  frame #1 {
                    n607 = global read "Trav_pos_global.vi" "Traverses to Move"() -> (w1036:string[])
                    n608 = global read "Constants_global.vi" "Traverse folder"() -> (w1037:path)
                    n609 = Strip Path(path=w1038) -> (stripped path=w1035:path)  [unwired: 1 out]
                    n610 = for {
                      tunnel: w1037 -> [w1050]
                      tunnel: w1036 -> [w1046] mode=indexing
                      tunnel: w1035 -> [w1047]
                      tunnel: string[] ["Traverse_Preferences.txt", "Traverse_Setup.xls"] ("Traverses to Move") -> [w1039]
                      n611 = Build Path(base path=w1050, name or relative path=w1046) -> (appended path=w1042:path)
                      n612 = Build Path(base path=w1042, name or relative path="Trav_Space_Files" ("Substring")) -> (appended path=w1049:path)
                      n613 = Build Path(base path=w1049, name or relative path="Selected_Filename.txt" ("Substring")) -> (appended path=w1054:path)
                      n614 = call "Create_directory_path.vi"("Path name"=w1054) -> ("Path name Out"=w1053:path)  [unwired: 1 in, 1 out]
                      n615 = Build Path(base path=w1047, name or relative path=w1046) -> (appended path=w1041:path)
                      n616 = for {
                        tunnel: w1042 -> [w1061]
                        tunnel: w1041 -> [w1059]
                        tunnel: w1039 -> [w1057] mode=indexing
                        n617 = Build Path(base path=w1061, name or relative path=w1057) -> (appended path=w1060:path)
                        n618 = Build Path(base path=w1059, name or relative path=w1057) -> (appended path=w1056:path)
                        n619 = call "Create_directory_path.vi"("Path name"=w1056) -> ("Path name Out"=w1055:path)  [unwired: 1 in, 1 out]
                        n620 = Copy(9:TRUE ("overwrite (F)"), 10:w1055, 11:w1060) -> ()  [unwired: 2 in, 3 out]
                      }
                      n621 = call "Read_File_Simple.vi"("Filename"=w1053) -> ("string"=w1044:string)  [unwired: 2 in, 7 out]
                      n622 = Build Path(base path=w1041, name or relative path=w1044) -> (appended path=w1045:path)
                      n623 = Build Path(base path=w1049, name or relative path=w1044) -> (appended path=w1048:path)
                      n624 = call "Create_directory_path.vi"("Path name"=w1045) -> ("Path name Out"=w1043:path)  [unwired: 1 in, 1 out]
                      n625 = Copy(9:TRUE ("overwrite (F)"), 10:w1043, 11:w1048) -> ()  [unwired: 2 in, 3 out]
                    }
                  }
                }
              }
            }
          }
        }
      }
      frame #20 {
        n626 = local read "Correlate?"() -> (w1066:T9)
        n627 = case shown="\"Run Program\"" w1063 {
          tunnel: w1063 -> [w1068 _ _ _]
          tunnel: [w1068 w1081 w1082 w1083] -> w1062
          frame "Run Program" {
            n628 = global read "Meas_global.vi" "Analysis Info cluster"() -> (w1067:T22[])
            n629 = for {
              tunnel: w1067 -> [w1079] mode=indexing
              stop <- w1069 stop-if-true
              w1076 = "Pitot ("
              n630 = Unbundle By Name(w1079) -> ("U"=w1070:dbl, "Inst name"=w1075:string)
              n631 = String Length(string=w1076) -> (length=w1078:i32)
              n632 = String Subset(string=w1075, length (rest)=w1078) -> (substring=w1077:string)  [unwired: 1 out]
              n633 = Equal?(x=w1077, y=w1076) -> (x = y?=w1072:bool)
              n634 = call "Match_Pat_Case_In.vi"("String to match"="ref", "String"=w1075) -> ("offset past match"=w1073:i32)  [unwired: 1 in, 3 out]
              n635 = Greater Or Equal To 0?(x=w1073) -> (x >= 0?=w1071:bool)
              n636 = And(x=w1071, y=w1072) -> (x .and. y?=w1069:bool)
              n637 = case shown="True" w1069 {
                tunnel: w1070 -> [_ w1080]
                frame False {
                }
                frame True {
                  n638 = call "Log_Reference_Velocity.vi"("Measured Velocity"=w1080) -> ()  [unwired: 1 out]
                }
              }
            }
          }
          frame "Show Setup" {
            w1081 = Setup."Run Program"  # setup
          }
          frame "Save Current Setup" {
            w1082 = Setup."Run Program"  # setup
          }
          frame "Setup Front Panel" {
            w1083 = Setup."Run Program"  # setup
          }
        }
        n639 = case shown="\"Correlate without activating panel\"" w1066 {
          tunnel: [T9."Cross correlation off" T9."Correlate without activating panel" T9."Correlate without activating panel"] -> w1065
          frame "Cross correlation off" {
          }
          frame "Show correlation panel" {
          }
          frame "Correlate without activating panel" {
          }
        }
        n640 = local write "Correlate?"(w1065) -> ()
        n641 = global write "Meas_global.vi" "Remote control"(FALSE ("Remote control")) -> ()
        n642 = call "Program_Active.vi"() -> ()  [unwired: 1 in]
        n643 = local write "setup"(w1062) -> ()
      }
      frame #21 {
        w1092 = FALSE  # Dialog Box (T)
        n644 = global read "Meas_global.vi" "Post Process"() -> (w1087:T2)
        n645 = case shown="\"Take New Data\"" w1087 {
          frame "Take New Data" {
            n646 = global read "Meas_global.vi" "Analysis Info cluster"() -> (w1104:T22[])
            n647 = global read "Meas_global.vi" "Requested Sampling rate"() -> (w1103:dbl)
            n648 = Divide(x=w1103, y=10.0) -> (x/y=w1096:dbl)
            n649 = Max & Min(x=w1096, y=100.0) -> (min(x,y)=w1095:dbl)  [unwired: 1 out]
            n650 = for {
              tunnel: w1104 -> [w1131] mode=indexing
              tunnel: w1095 -> [w1125]
              tunnel: [w1127] -> w1101
              tunnel: [w1126] -> w1099
              tunnel: [w1124] -> w1098
              stop <- w1127 stop-if-true
              n651 = Unbundle By Name(w1131) -> ("Inst name"=w1126:string, "Av Sampling Rate"=w1124:dbl, "Inst type"=w1130:T16)
              n652 = Equal?(x=w1130, y=Inst_type."LDA Vel" ("Inst type")) -> (x = y?=w1128:bool)
              n653 = Less?(x=w1124, y=w1125) -> (x < y?=w1123:bool)
              n654 = Greater Than 0?(x=w1124) -> (x > 0?=w1122:bool)
              n655 = Compound Arithmetic op=AND(w1123, w1122, w1128) -> (w1127:bool)
            }
            n656 = case shown="True" w1101 {
              tunnel: [FALSE w1106] -> w1100
              frame False {
              }
              frame True {
                n657 = global read "Preference_global.vi" "Rig Setup"() -> (w1112:string)
                n658 = Concatenate Strings("Status:of:", w1112) -> (w1111:string)
                n659 = Build Array(w1111) -> (w1110:string[])
                n660 = call "Get_Current_Scan_client.vi"("ADAM Ch Names"=w1110) -> ("Numerical Values"=w1109:dbl[])  [unwired: 1 in, 2 out]
                n661 = Index Array(array=w1109) -> (element=w1108:dbl)  [unwired: 1 in]
                n662 = Equal?(x=2.0, y=w1108) -> (x = y?=w1106:bool)
              }
            }
            n663 = case shown="True" w1100 {
              tunnel: w1099 -> [_ w1117]
              tunnel: w1098 -> [_ w1115]
              frame False {
              }
              frame True {
                w1120 = FALSE  # Dialog Box (T)
                n664 = Format Into String(format string="The %s currently has a data rate of %d Hz", w1117, w1115) -> (resulting string=w1116:string)  [unwired: 2 in, 1 out]
                n665 = Bundle By Name(cluster=errorcluster {"status"=TRUE, "code"=0, "source"=""} ("error in (no error)"), "source"=w1116) -> (w1119:errorcluster)
                n666 = call "EnFlo_Error_Handler.vi"("error in (no error)"=w1119, "Error Type"="Low LDA Sampling Rate", "Dialog Box (T)"=w1120) -> ()  [unwired: 3 out]
              }
            }
          }
          frame "Post Process Raw Data File" {
          }
        }
        n667 = global read "Meas_global.vi" "Over/Under string"() -> (w1090:string)
        n668 = Empty String/Path?(string/path=w1090) -> (empty?=w1089:bool)
        n669 = Not(x=w1089) -> (.not. x?=w1088:bool)
        n670 = Bundle By Name(cluster=errorcluster {"status"=FALSE, "code"=0, "source"=""} ("error in (no error)"), "source"=w1090, "status"=w1088) -> (w1093:errorcluster)
        n671 = call "EnFlo_Error_Handler.vi"("error in (no error)"=w1093, "Error Type"="Signal Clipping", "Dialog Box (T)"=w1092) -> ()  [unwired: 3 out]
      }
      frame #22 {
        w1134 = string[] [] ("Per Block Plug Ins Extra")
        n672 = Empty String/Path?(string/path=w1138) -> (empty?=w1137:bool)
        n673 = global read "Dynamic_call_global.ph.vi" "Final Plug Ins"() -> (w1139:string[])
        n674 = case shown="True" w1137 {
          tunnel: w1138 -> [w1150 _]
          frame False {
            n675 = local read "Comments"() -> (w1149:string)
            n676 = call "Fast_string_Replace.vi"("Replace match with:"="", "Input String"=w1149, "regular expression"=w1150) -> ("Output String"=w1148:string)  [unwired: 2 out]
            n677 = local write "Comments"(w1148) -> ()
          }
          frame True {
          }
        }
        n678 = call "Plug_in_Directories.vi"() -> ("Final"=w1135:path)  [unwired: 3 out]
        n679 = for {
          tunnel: w1139 -> [w1153] mode=indexing
          tunnel: w1135 -> [w1152]
          w1156 = FALSE  # Dialog Box (T)
          n680 = Build Path(base path=w1152, name or relative path=w1153) -> (appended path=w1151:path)
          n681 = global read "Dynamic_call_global.ph.vi" "Plug in"() -> (w1161:refnum<vi>)
          n682 = Open VI Reference(type specifier VI Refnum (for type only)=w1161, vi path=w1151) -> (vi reference=w1160:refnum<vi>, error out=w1159:errorcluster)  [unwired: 2 in, 2 out]
          n683 = call-by-ref "?"(reference=w1160, error in=w1159) -> (reference out=w1157:refnum<vi>, error out=w1158:errorcluster)  [unwired: 6 in, 2 out]
          n684 = Close Reference(reference=w1157, error in (no error)=w1158) -> (error out=w1154:errorcluster)
          n685 = call "EnFlo_Error_Handler.vi"("error in (no error)"=w1154, "Error Type"="Running Final Plug In", "Dialog Box (T)"=w1156) -> ()  [unwired: 3 out]
        }
        n686 = global read "Meas_global.vi" "Repeat Measurement?"() -> (w1136:bool)
        n687 = case shown="True" w1136 {
          tunnel: w1133 -> [_ w1146]
          tunnel: [FALSE w1141] -> w1132
          frame False {
          }
          frame True {
            n688 = global read "Meas_global.vi" "Post Process"() -> (w1144:T2)
            n689 = Equal To 0?(x=w1146) -> (x = 0?=w1142:bool)
            n690 = Equal?(x=w1144, y=Post_Process."Post Process Raw Data File" ("Post Process")) -> (x = y?=w1143:bool)
            n691 = And(x=w1143, y=w1142) -> (x .and. y?=w1141:bool)
          }
        }
        n692 = global write "Dynamic_call_global.ph.vi" "Per Block Plug Ins Extra"(w1134) -> ()
        n693 = global write "Dynamic_call_global.ph.vi" "Initial Plug Ins Extra"(w1134) -> ()
      }
      frame #23 {
        n694 = global read "Meas_global.vi" "Post Process"() -> (w1168:T2)
        n695 = local read "stop"() -> (w1174:bool)
        n696 = Equal?(x=w1169, y=Setup."Run Program" ("setup")) -> (x = y?=w1165:bool)
        n697 = Equal?(x=w1168, y=Post_Process."Take New Data" ("Post Process")) -> (x = y?=w1166:bool)
        n698 = And(x=w1165, y=w1166) -> (x .and. y?=w1164:bool)
        n699 = case shown="False" w1174 {
          tunnel: [Multi_Run_Status."Continue" ("Status Out") Multi_Run_Status."Terminate Run" ("Status Out")] -> w1172
          frame False {
          }
          frame True {
            n700 = local write "stop"(FALSE) -> ()
          }
        }
        n701 = case shown="True" w1164 {
          tunnel: w1172 -> [w1175 w1179]
          tunnel: [w1175 w1181] -> w1171
          frame False {
          }
          frame True {
            n702 = local read "Raw data file"() -> (w1180:path)
            n703 = global read "Meas_global.vi" "Acquisition vi Ref"() -> (w1176:refnum<vi>)
            n704 = Path to Array of Strings(0:w1180) -> (2:w1182:string[])  [unwired: 1 out]
            n705 = Index Array(array=w1182, index=0 ("Index")) -> (element=w1178:string)
            n706 = Close Reference(reference=w1176) -> ()  [unwired: 1 in, 1 out]
            n707 = Build Array(w1178) -> (w1177:string[])
            n708 = for {
              tunnel: w1177 -> [w1186] mode=indexing
              shift-right: [w1184] -> w1181
              shift-left: w1179 -> [w1185]
              n709 = call "Warn_on_low_HD_space.vi"("Status In"=w1185, "HD name"=w1186) -> ("Status Out"=w1184:T1)  [unwired: 6 out]
            }
          }
        }
        "Status Out" <- w1171
        n710 = global write "Trav_pos_global.vi" "Dummy Measurement?"(FALSE ("Dummy Measurement?")) -> ()
        n711 = global write "Plug_in_data_global.vi" "Server Channels to log"(string[] [] ("Server Channels to log")) -> ()
        n712 = global write "Meas_global.vi" "Extra Comments"("") -> ()
      }
    }
  }
